vi "TL24 Tool Main.vi"() -> ()   [LabVIEW 2016]
uses:
  Common/LabVIEW GEA2 Toolkit/LabVIEW_GEA2_Toolkit.lvlibp/type defs/Data In.ctl
  Common/LabVIEW GEA2 Toolkit/LabVIEW_GEA2_Toolkit.lvlibp/type defs/Source_Destination.ctl
  Common/LabVIEW GEA2 Toolkit/LabVIEW_GEA2_Toolkit.lvlibp/type defs/Data Type.ctl
  Common/LabVIEW GEA2 Toolkit/LabVIEW_GEA2_Toolkit.lvlibp/type defs/ERD Read Data In.ctl
  Laundry Tool 2.0 Support/type defs2/Select _Graph_Brass.ctl
  Laundry Tool 1.0 Support/type defs/ERD_Graph_All.ctl
  Laundry Tool 1.0 Support/type defs/ERD_Graph.ctl
  Laundry Tool 1.0 Support/type defs/Version.ctl
  Laundry Tool 2.0 Support/type defs2/ERD_Always_Show_Brass.ctl
  Laundry Tool 1.0 Support/type defs/Fault_Buffer_Status.ctl
  Laundry Tool 2.0 Support/type defs2/Diagnostics_Table.ctl
  Laundry Tool 1.0 Support/type defs/Cycle_Diag_Buffer_Status.ctl
  Laundry Tool 2.0 Support/type defs2/ERD_Data_Loop_Control_Brass.ctl
  Laundry Tool 2.0 Support/type defs2/ERD_Loop_States_Brass.ctl
  Laundry Tool 2.0 Support/type defs2/Error_Command_Brass.ctl
  Laundry Tool 2.0 Support/type defs2/DAQ_States_Brass.ctl
  Common/GExplorer Support/typedefs/GExplorer_Data_Cluster.ctl
  Laundry Tool 1.0 Support/type defs/Cont_Send_States.ctl
  Laundry Tool 2.0 Support/type defs2/Cont_Send_States_Brass.ctl
  Common/LabVIEW GEA2 Toolkit/LabVIEW_GEA2_Toolkit.lvlibp/type defs/Data Out.ctl
  Common/LabVIEW GEA2 Toolkit/LabVIEW_GEA2_Toolkit.lvlibp/type defs/ERD Write Data In.ctl
  Laundry Tool 2.0 Support/type defs2/DAQ_Control_Command_Brass.ctl
  Laundry Tool 2.0 Support/type defs2/ERD_Loop_Control_Command_Brass.ctl
  Laundry Tool 2.0 Support/type defs2/GEA2_Control_Command_Brass.ctl
  <vilib>/DAQmx/read.llb/DAQmx Read (Digital 1D Bool NChan 1Samp 1Line).vi
  <vilib>/DAQmx/read.llb/DAQmx Read (Digital 1D U8 1Chan NSamp).vi
  <vilib>/DAQmx/write.llb/DAQmx Write (Digital Bool 1Line 1Point).vi
  <vilib>/DAQmx/read.llb/DAQmx Read (Counter U32 1Chan 1Samp).vi
  <vilib>/DAQmx/write.llb/DAQmx Write (Analog 1D DBL NChan 1Samp).vi
  <vilib>/DAQmx/write.llb/DAQmx Write (Digital 1D Bool NChan 1Samp 1Line).vi
  Common/LabVIEW GEA2 Toolkit/LabVIEW_GEA2_Toolkit.lvlibp/advanced/GEA2 Message Received Event Handler.vi
  <vilib>/DAQmx/create/channels.llb/DAQmx Create Channel (DO-Digital Output).vi
  <vilib>/DAQmx/create/channels.llb/DAQmx Create Channel (DI-Digital Input).vi
  <vilib>/DAQmx/configure/timing.llb/DAQmx Timing (Sample Clock).vi
  <vilib>/DAQmx/create/channels.llb/DAQmx Create Channel (CO-Pulse Generation-Frequency).vi
  <vilib>/DAQmx/configure/timing.llb/DAQmx Timing (Implicit).vi
  <vilib>/DAQmx/create/channels.llb/DAQmx Create Channel (CI-Count Edges).vi
  <vilib>/DAQmx/create/channels.llb/DAQmx Create Channel (AO-Voltage-Basic).vi
  <vilib>/DAQmx/miscellaneous.llb/DAQmx Fill In Error Info.vi
  C:/Automation/DLLs/PC Dot Net/GeaCommunication.dll
  Common/LabVIEW GEA2 Toolkit/LabVIEW_GEA2_Toolkit.lvlibp
  Automation/Product Specific/Clothes Care/2015 VA Washer/Projects/2015 VA Washer.lvlib
  <resource>/objmgr/daqmx.rc
panel:
  in  "Data ON":bool=TRUE
  out "ERD_Always Show":T1
  in  "Stop":bool
  out "Fault Status":bool
  out "Log Rate (ms)":u32
  in  "Tab Control":T2(tab)
  in  "Filter Data":bool=TRUE
  in  "Start Send":bool
  in  "Cmd":string
  in  "Filter Log":bool
  in  "Msg Rate (ms)":u32=1000 min=50 step=50
  out "CSV File Log Path":path=path "C:/Users/502129737/Desktop/1"
  in  "Clear":bool
  out "GEA2 Log":string
  in  "Board Index":u8 max=0 step=1
  out "Board ID":string="0"
  in  "GEA2 Send":T3={"Source"=228, "Destination"=50, "Command"=0, "Message"=""} {"Command" format="%02x"; "Destination" format="%02x"; "Source" format="%02x"}
  in  "Send Button":bool
  in  "GEA2 Log Length":i32=100000
  in  "Save Log":bool
  out "Version":T4
  in  "GEA Inputs":T5={"Source"=228, "Destination"=50} {"Destination" format="%.0x"; "Source" format="%.0x"}
  in  "Read ERD List":T6[](array[typedef])=[{"ERD Number"=0, "Data Type"=enum."string"}] {"ERD Number" format="%.0x"}
  out "Read ERD Data Out":cluster{"ERD Number":u16, "Data":string}[](array[cluster]) {"ERD Number" format="%.0x"}
  in  "Read ERD":bool
  in  "Write ERD":bool
  in  "Write ERD List":T8(array[cluster])=[{"ERD Number"=0, "Data Type"=enum."string", "Data"=""}] {"ERD Number" format="%.0x"}
  in  "ERD Graphing ON":bool
  out "ERD Graph  Ind":T9
  in  "ERD Graph Cntrl":T10={"ERD 3"={"ERD #"=62250, "Data Type"=enum."uint16_t", "Scaler"=32}, "ERD 2"={"ERD #"=62250, "Data Type"=enum."uint16_t", "Scaler"=32}, "ERD 1"={"ERD #"=62250, "Data Type"=enum."uint16_t", "Scaler"=32}} {"ERD 1"."Scaler" min=1; "ERD 1"."ERD #" format="%.0x"; "ERD 2"."Scaler" min=1; "ERD 2"."ERD #" format="%.0x"; "ERD 3"."Scaler" min=1; "ERD 3"."ERD #" format="%.0x"}
  in  "Graphing ON":bool=TRUE
  in  "Select Graph":T12=enum."All Loads"
  out "ERD 3":dbl(graph)
  out "ERD 2":dbl(graph)
  out "ERD 1":dbl(graph)
  in  "Save Fault Log":bool
  in  "Clear Fault Table Buffer":bool
  in  "Clear Fault Seq Buffer":bool
  in  "Fault ON":bool
  out "Fault Table Buffer":string[][](table)
  out "Fault Sequence Buffer":string
  out "Seq Buffer Status":T13
  out "Table Buffer Status":T13
  in  "Save Cycle History Log":bool
  in  "Clear Cycle Buffer":bool
  out "Cycle Buffer Status":T14
  in  "Get Cycle History":bool
  out "Diagnostics Table":T15
  in  "HE/LE ?":enum16{"HE", "LE"}(ring)
  in  "LL (M - A)":bool=TRUE
  in  "Lid Lock Feedback":bool
  in  "MS (M - A)":bool=TRUE
  out "DAQ Status":string
  out "Drain Pump":bool
  out "Mode Shift":bool
  out "Recirc Pump":bool
  out "Cold Valve":bool
  out "Hot Valve":bool
  out "Spray/Rinse Valve":bool
  out "Fabric SoftValve":bool
  in  "AC Power":bool=TRUE
  in  "Mode Shift FB":bool
  in  "Lid Status":bool=TRUE
  in  "Pressure":dbl(slide) min=0.0 max=5.0 step=0.5 scale=0.0..5.0 scale format="%#_3g"
  in  "Motor Current":dbl(slide)=2.5 min=0.0 max=5.0 step=0.5 scale=0.0..5.0 scale format="%#_3g"
  in  "Turn On DAQ":bool
  out "DAQ On?":bool
  in  "Basket RPM":dbl=1.0 min=1.0 max=800.0 step=5.0
  in  "Temperature":dbl(slide)=2.5 min=0.0 max=5.0 step=0.5 scale=0.0..5.0 scale format="%#_3g"
  out "Triac CW":bool
  out "Traic CCW":bool
  out "CCW":u32
  out "CW":u32
  in  "ERD Read List":T16(array[cluster])=[{"Boolean"=TRUE, "ERD Number"=1, "ERD Name"="Model Number", "Data Type"=enum."string"}, {"Boolean"=TRUE, "ERD Number"=2, "ERD Name"="Serial Number", "Data Type"=enum."string"}, {"Boolean"=TRUE, "ERD Number"=8192, "ERD Name"="Machine Status", "Data Type"=enum."uint8_t"}, {"Boolean"=TRUE, "ERD Number"=8202, "ERD Name"="Cycle Name", "Data Type"=enum."string"}, {"Boolean"=TRUE, "ERD Number"=8213, "ERD Name"="Soil Level", "Data Type"=enum."string"}, {"Boolean"=TRUE, "ERD Number"=142, "ERD Name"="Cycle Count", "Data Type"=enum."uint32_t"}, {"Boolean"=TRUE, "ERD Number"=8193, "ERD Name"="Sub-Cycle", "Data Type"=enum."string"}, {"Boolean"=TRUE, "ERD Number"=141, "ERD Name"="System Runtime", "Data Type"=enum."uint32_t"}, {"Boolean"=TRUE, "ERD Number"=8208, "ERD Name"="Delay Time", "Data Type"=enum."uint16_t"}, {"Boolean"=TRUE, "ERD Number"=256, "ERD Name"="Version", "Data Type"=enum."string"}, {"Boolean"=TRUE, "ERD Number"=70, "ERD Name"="Cycle Time", "Data Type"=enum."uint16_t"}, {"Boolean"=TRUE, "ERD Number"=8206, "ERD Name"="Operating Mode", "Data Type"=enum."string"}, {"Boolean"=TRUE, "ERD Number"=8214, "ERD Name"="Temp Level", "Data Type"=enum."uint8_t"}, {"Boolean"=TRUE, "ERD Number"=8215, "ERD Name"="Spin Level", "Data Type"=enum."uint8_t"}, {"Boolean"=TRUE, "ERD Number"=61440, "ERD Name"="Water Level", "Data Type"=enum."uint8_t"}, {"Boolean"=TRUE, "ERD Number"=8216, "ERD Name"="Rinse Option", "Data Type"=enum."uint8_t"}] {"ERD Number" format="%.0x"}
  out "Error Out":errorcluster
  in  "Error In":errorcluster
  # "Software Version"
  # "UI"
  # "MC"
  # "Must input a valid ERD# and Data Type\nDO NOT Leave Blank \nIf no scaler use value of 01"
  # "Contact:\n\nDerek Hibdon\nderek.hibdon@ge.com"
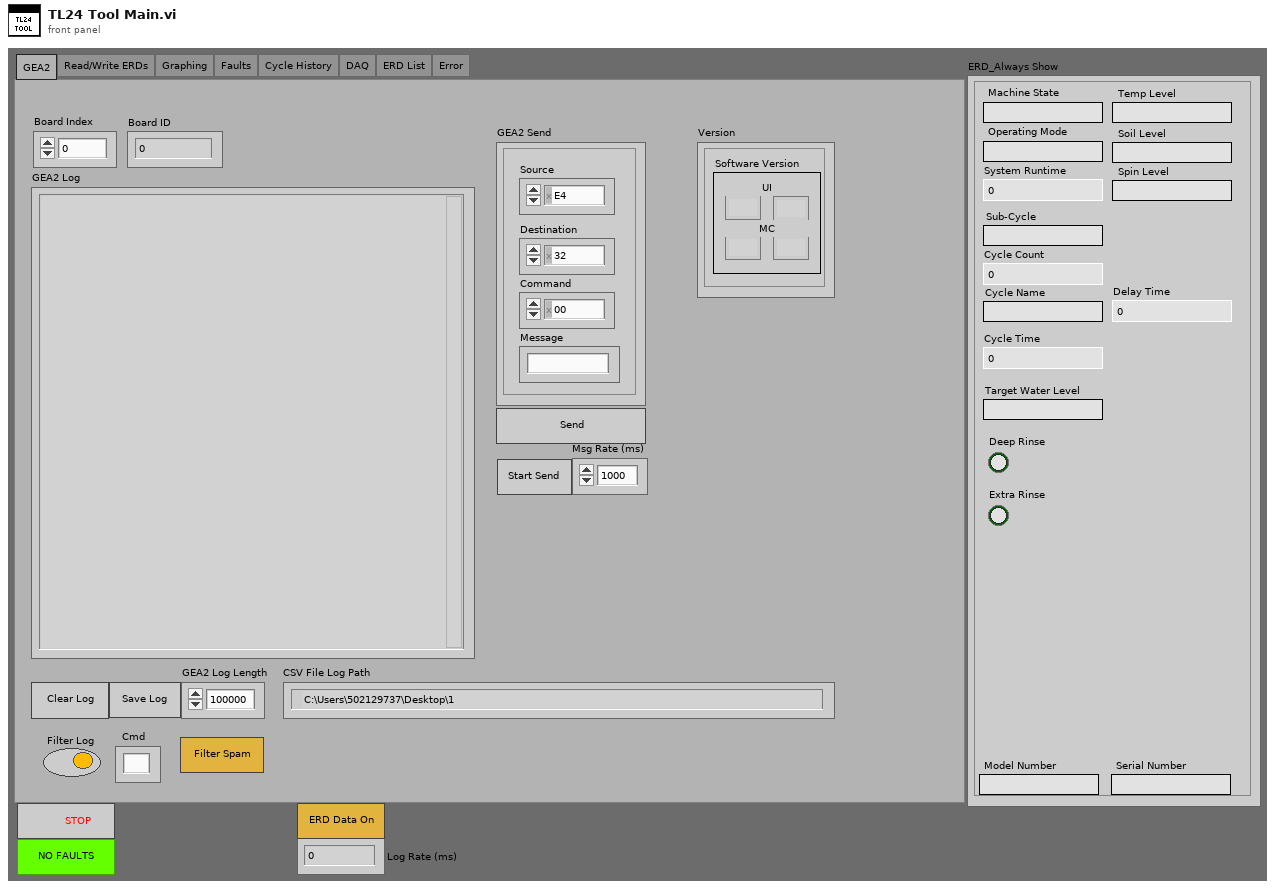
[diagram p1: front panel]
types:
  T1 = typedef "ERD_Always_Show_Brass.ctl" = cluster{"Machine State":string, "Cycle Count":u32, "Soil Level":string, "Spin Level":string, "Temp Level":string, "Delay Time":u16, "Sub-Cycle":string, "Cycle Name":string, "Model Number":string, "Serial Number":string, "System Runtime":u32, "Cycle Time":u16, "Operating Mode":string, "Target Water Level":string, "Deep Rinse":bool, "Extra Rinse":bool}
  T2 = enum32{"GEA2", "Read/Write ERDs", "Graphing", "Faults", "Cycle History", "DAQ", "ERD List", "Error"}
  T3 = typedef "LabVIEW_GEA2_Toolkit.lvlibp/Data In.ctl" = cluster{"Source":u8, "Destination":u8, "Command":u8, "Message":string}
  T4 = typedef "Version.ctl" = cluster{"Critical Major":string, "Critical Minor":string, "Non-Critical Minor":string, "Non-Critical Major":string}
  T5 = typedef "LabVIEW_GEA2_Toolkit.lvlibp/Source_Destination.ctl" = cluster{"Source":u8, "Destination":u8}
  T6 = typedef "LabVIEW_GEA2_Toolkit.lvlibp/ERD Read Data In.ctl" = cluster{"ERD Number":u16, "Data Type":T7}
  T7 = typedef "LabVIEW_GEA2_Toolkit.lvlibp/Data Type.ctl" = enum16{"string", "boolean", "uint8_t", "uint16_t", "uint32_t", "uint64_t", "int8_t", "int16_t", "int32_t", "int64_t"}
  T8 = cluster{"ERD Number":u16, "Data Type":T7, "Data":string}[]
  T9 = cluster{"ERD Value 1":dbl, "ERD Value 2":dbl, "ERD Value 3":dbl}
  T10 = typedef "ERD_Graph_All.ctl" = cluster{"ERD 3":T11, "ERD 2":T11, "ERD 1":T11}
  T11 = typedef "ERD_Graph.ctl" = cluster{"ERD #":u16, "Data Type":T7, "Scaler":u32}
  T12 = typedef "Select _Graph_Brass.ctl" = enum16{"Temperature (F)", "Basket Speed (RPM)", "Tub Volume (Gal)", "Pressure (in H2O)", "Current RMS (Amps)", "ERD 1", "ERD 2", "ERD 3", "All Loads"}
  T13 = typedef "Fault_Buffer_Status.ctl" = cluster{"Current Index":u16, "Count":u16, "Overwrite Count":u16}
  T14 = typedef "Cycle_Diag_Buffer_Status.ctl" = cluster{"Current Index":u16, "Count":u16, "Overwrite Count":u16}
  T15 = typedef "Diagnostics_Table.ctl" = string[][]
  T16 = cluster{"Boolean":bool, "ERD Number":u16, "ERD Name":string, "Data Type":enum16{"string", "boolean", "uint8_t", "uint16_t", "uint32_t", "uint64_t"}}[]
  T17 = typedef "Cont_Send_States_Brass.ctl" = enum16{"Run", "Shutdown"}
  T18 = typedef "Cont_Send_States.ctl" = enum16{"Run", "Shutdown"}
  T19 = typedef "GExplorer_Data_Cluster.ctl" = cluster{"Data":variant, "State":enum16{"Add to Log", "Clear", "Shutdown"}}
  T20 = typedef "DAQ_States_Brass.ctl" = enum16{"Wait for Init", "Rename Devices", "Verify Hardware", "Initialize", "Run", "Shutdown", "Exit"}
  T21 = typedef "ERD_Data_Loop_Control_Brass.ctl" = cluster{"Data":variant, "State":T22}
  T22 = typedef "ERD_Loop_States_Brass.ctl" = enum16{"Init", "Build ERD Read List", "Read ERDs", "Update UI", "Update Graphs", "Read Faults", "Log Data", "Pause", "Shutdown"}
  T23 = typedef "Error_Command_Brass.ctl" = enum16{"Initialize", "Handle Errors", "Report Errors"}
  T24 = typedef "LabVIEW_GEA2_Toolkit.lvlibp/ERD Write Data In.ctl" = cluster{"ERD Number":u16, "Data Type":T7, "Data":string}
  T25 = typedef "GEA2_Control_Command_Brass.ctl" = enum16{"Initialize", "Shutdown"}
  T26 = typedef "ERD_Loop_Control_Command_Brass.ctl" = enum16{"Initialize", "Shutdown"}
  T27 = typedef "DAQ_Control_Command_Brass.ctl" = enum16{"Initialize", "Shutdown", "Exit"}
  T28 = enum8{"Enabled", "Disabled", "Disabled and Grayed Out"}
  T29 = typedef "LabVIEW_GEA2_Toolkit.lvlibp/Data Out.ctl" = cluster{"Source":u8, "Destination":u8, "Command":u8, "Length":u8, "CRC":u16, "Message":string}
  T30 = typedef "LabVIEW_GEA2_Toolkit.lvlibp/ERD Read Data Out.ctl" = cluster{"ERD Number":u16, "Data":string}
  T31 = typedef "All_Bundled_Data_Brass.ctl" = cluster{"Version":T4, "ERD_Always Show":T1, "Personality Set":u8, "CSV File String Arrays":T32, "Fault Table Array ":T33}
  T32 = typedef "CSV_File_String_Arrays.ctl" = cluster{"ERD Number Array":string[], "ERD Name Array":string[], "ERD Converted String Data":string[]}
  T33 = typedef "Fault Table Array.ctl" = T34[]
  T34 = typedef "Fault_Table_Info.ctl" = cluster{"Cycle Count":u32, " Runtime (min) ":u32, "Fault Status":string, "Fault ID":string, "Fault Count":u16}
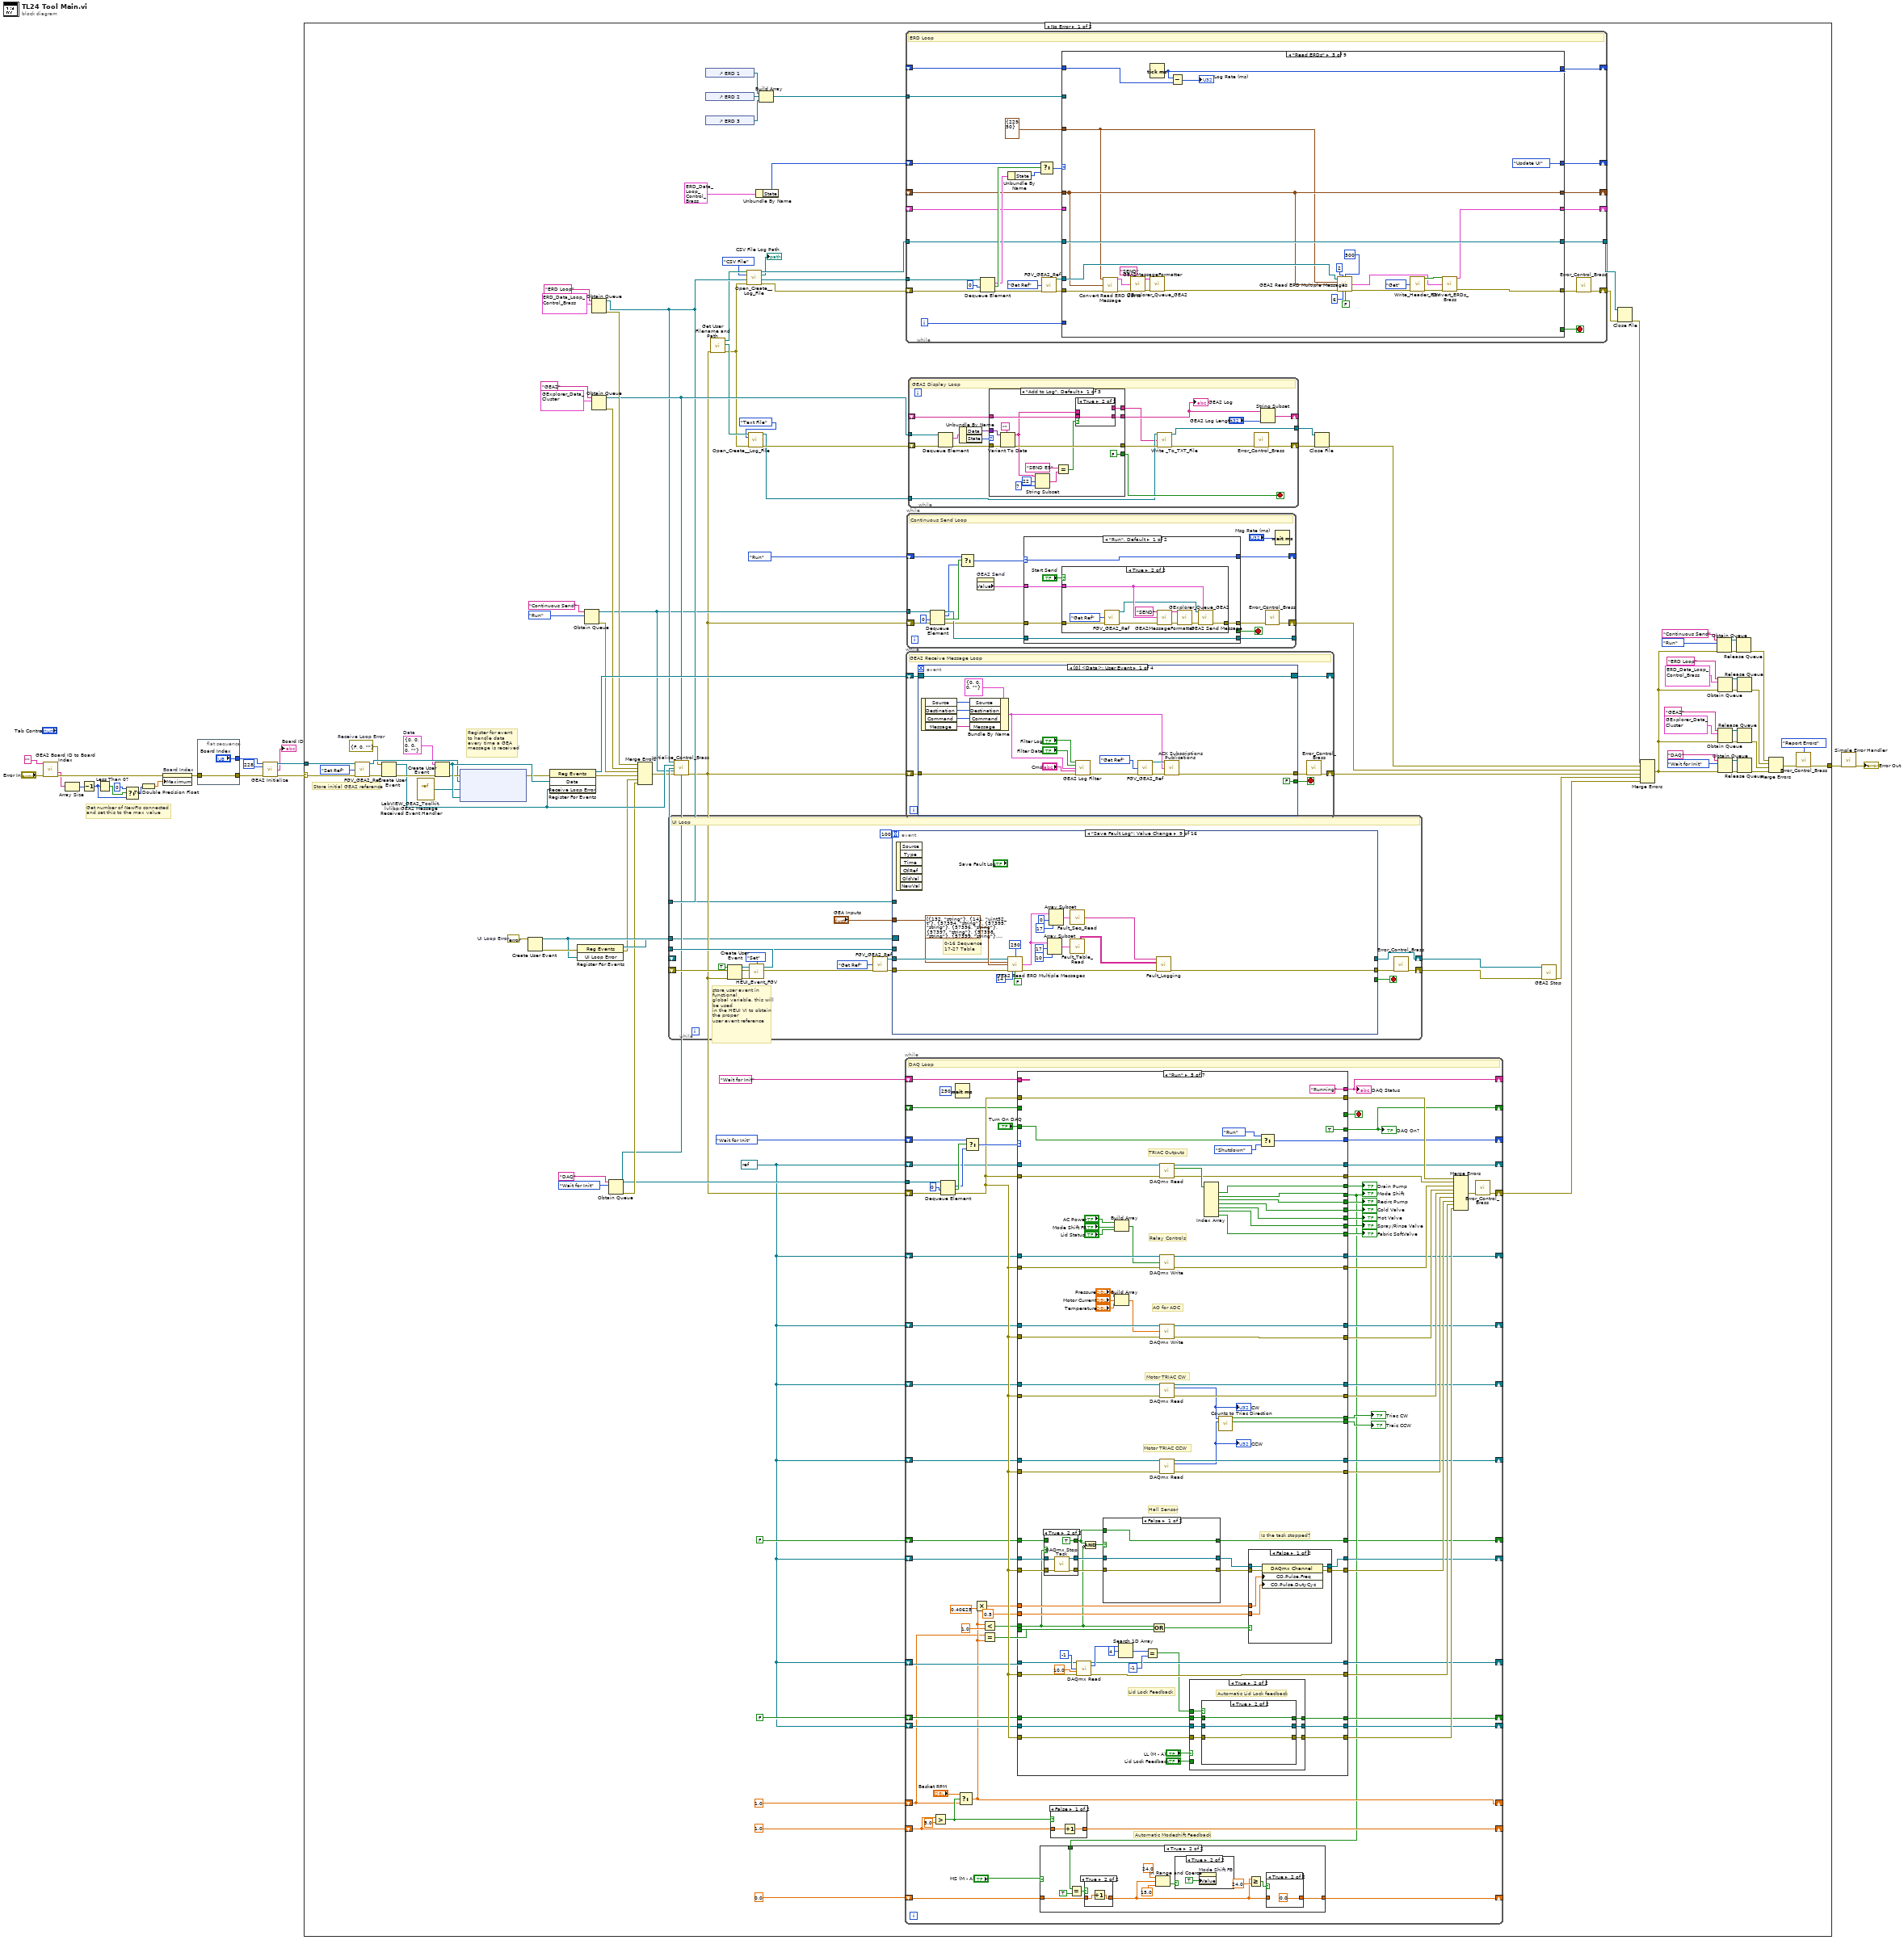
[diagram p0: block diagram]
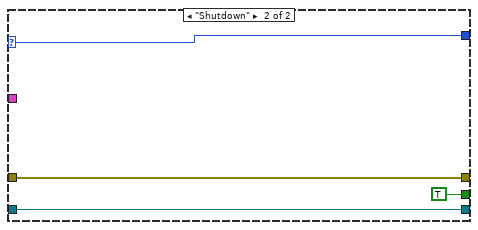
[diagram p3: hidden frame]
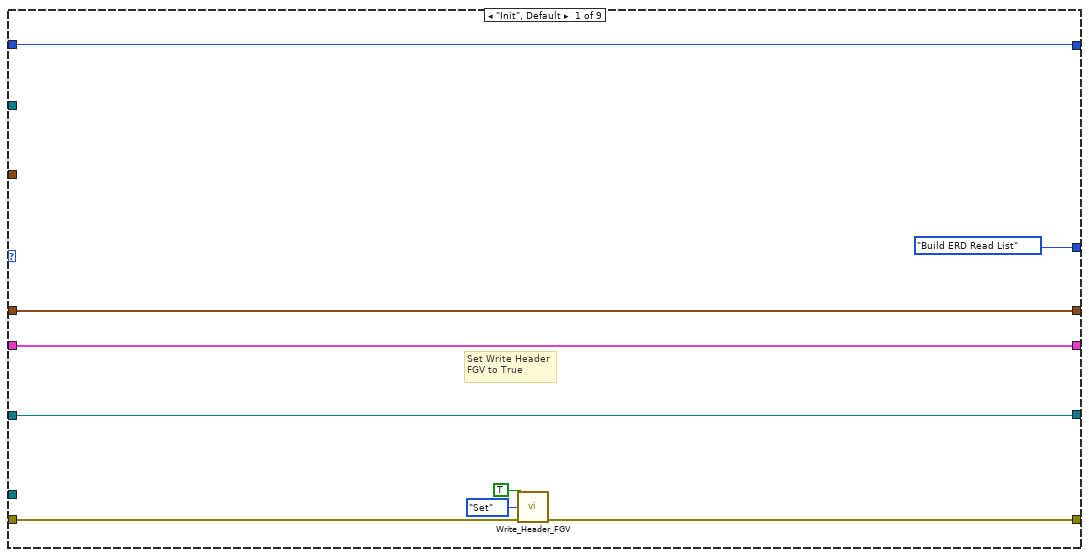
[diagram p4: hidden frame]
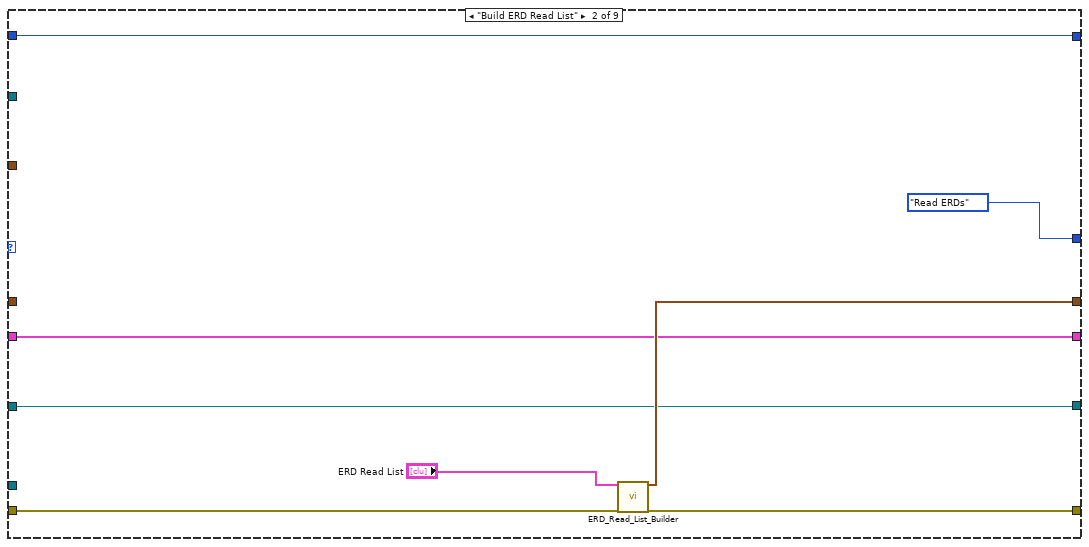
[diagram p5: hidden frame]
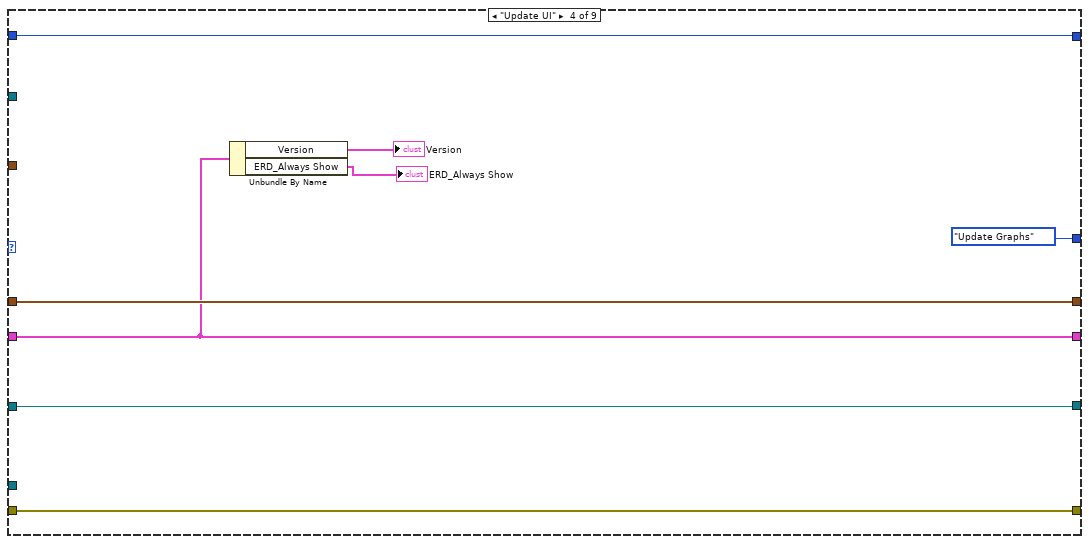
[diagram p6: hidden frame]
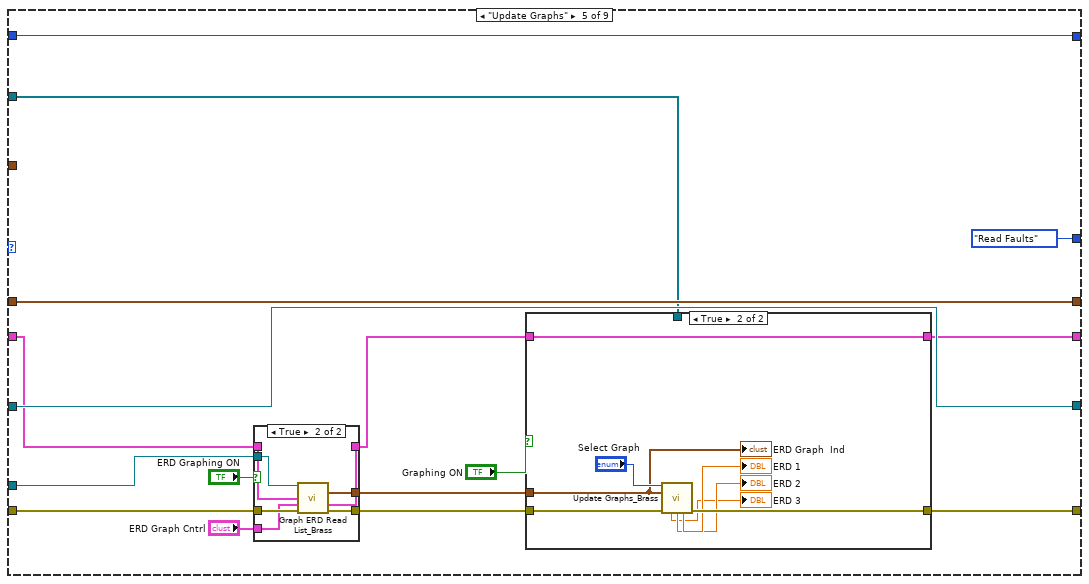
[diagram p7: hidden frame]
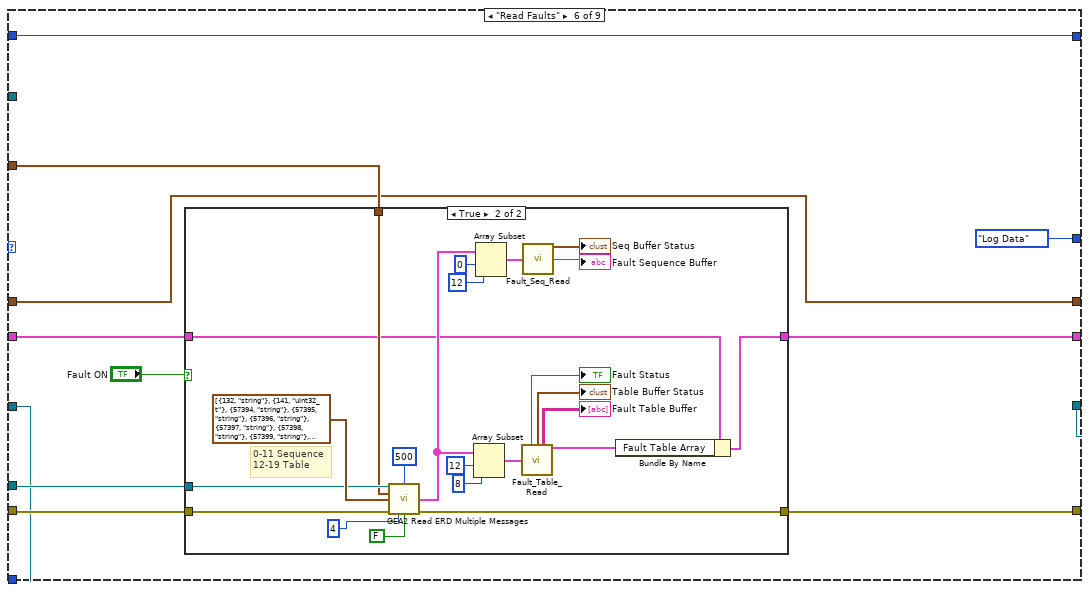
[diagram p10: hidden frame]
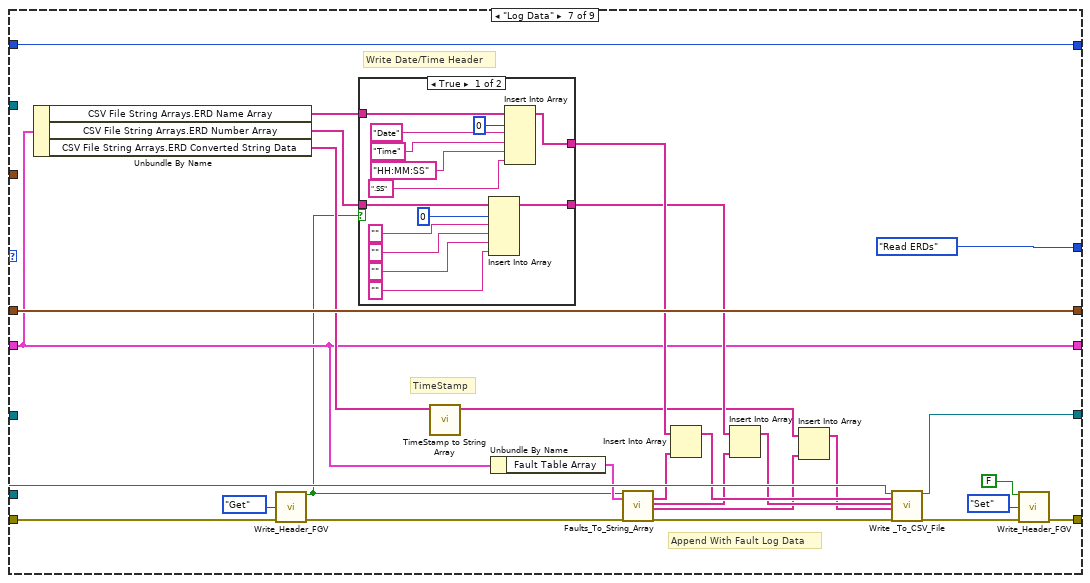
[diagram p12: hidden frame]
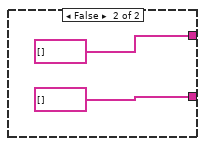
[diagram p13: hidden frame]
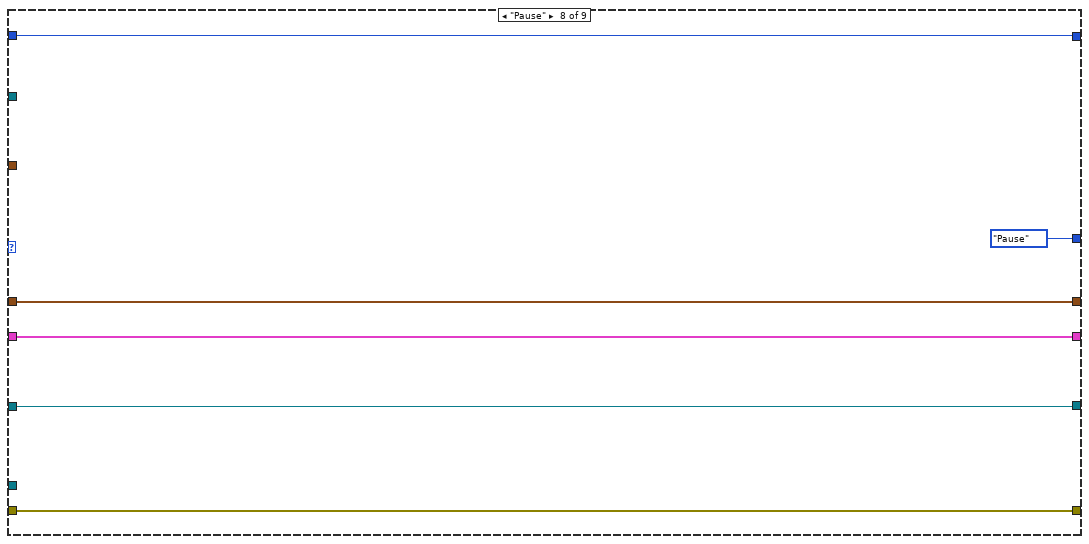
[diagram p14: hidden frame]
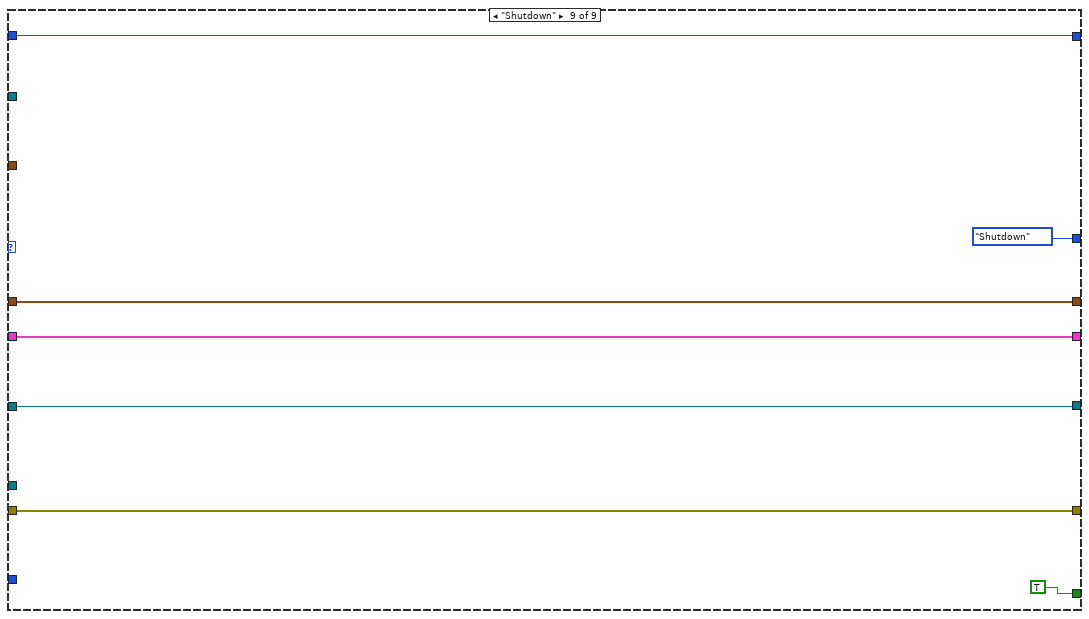
[diagram p15: hidden frame]
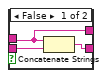
[diagram p16: hidden frame]
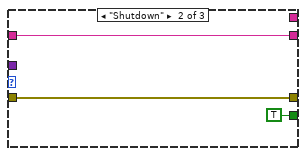
[diagram p17: hidden frame]
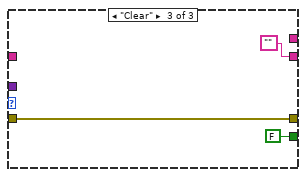
[diagram p18: hidden frame]
diagram:
  # "Get number of NewFIs connected\nand set this to the max value"
  n1 = call "GEA2 Board ID to Board Index.vi"("Board ID"="", "Error In"="Error In") -> ("Boards Found"=w4:string[], "Error Out"=w13:errorcluster)  [unwired: 9 in, 3 out]
  n2 = Array Size(array=w4) -> (size(s)=w9:i32)
  n3 = Decrement(x=w9) -> (x-1=w7:i32)
  n4 = Less Than 0?(x=w7) -> (x < 0?=w8:bool)
  n5 = Select(t=0, s=w8, f=w7) -> (s? t:f=w5:i32)
  n6 = To Double Precision Float(number=w5) -> (double precision float=w3:dbl)
  n7 = property on="Board Index" class="DigNum (strict)"(error in=w13, "Maximum"=w3) -> (error out=w11:errorcluster)  [unwired: 1 in, 1 out]
  n8 = flat-sequence {
    tunnel: ["Board Index"] -> w16
    tunnel: w11 -> [w20]
    tunnel: [w20] -> w10
    frame #0 {
    }
  }
  n9 = call "GEA2 Initialize.vi"("Board Index"=w16, "Source Address"=u8 228, "error in"=w10) -> ("GEA2 Reference Out"=w18:refnum<k24>, "Board ID"=→"Board ID":string, "error out"=w17:errorcluster)  [unwired: 10 in]
  n10 = case shown="No Error" w17 {
    selector: w17 -> [w80 w1258]
    tunnel: w18 -> [w78 _]
    tunnel: [w82 w1258] -> w2
    frame No Error {
      w34 = errorcluster {"status"=FALSE, "code"=0, "source"=""}  # Receive Loop Error
      w35 = T29 {"Source"=0, "Destination"=0, "Command"=0, "Length"=0, "CRC"=0, "Message"=""}  # Data
      w50 = refnum<k21> refnum ("task out")
      w116 = errorcluster {"status"=FALSE, "code"=0, "source"=""}  # UI Loop Error
      # "store user event in functional\nglobal variable, this will be used\nin the HEUI VI to obtain the proper\nuser event reference"
      # "Store initial GEA2 reference"
      # "Register for event\nto handle data\nevery time a GEA\nmessage is received"
      n11 = call "FGV_GEA2_Ref.vi"("GEA2 Reference In"=w78, "Action"=enum16{"Set Ref", "Get Ref"}."Set Ref", "Error In"=w80) -> ("GEA2 Reference Out"=w77:refnum<k24>, "Error Out"=w79:errorcluster)  [unwired: 11 in]
      n12 = Create User Event(user event datatype=w34, error in=w79) -> (user event=w117:refnum<user-event>, error out=w119:errorcluster)
      n13 = vi-ref "LabVIEW_GEA2_Toolkit.lvlibp:GEA2 Message Received Event Handler.vi"() -> (w118:refnum<vi>)
      n14 = Create User Event(user event datatype=w35, error in=w119) -> (user event=w122:refnum<user-event>, error out=w121:errorcluster)
      n15 = node(w121, w77, w118, w122) -> (w120:errorcluster)  [unwired: 1 in, 1 out]
      n16 = Create User Event(user event datatype=w116) -> (user event=w105:refnum<user-event>, error out=w115:errorcluster)  [unwired: 1 in]
      n17 = register-events(error in=w120, w122, w117) -> (reference out=w114:refnum<event-registration>, error out=w87:errorcluster)  [unwired: 1 in]
      n18 = register-events(error in=w115, w105) -> (reference out=w96:refnum<event-registration>, error out=w86:errorcluster)  [unwired: 1 in]
      n19 = Obtain Queue(name (unnamed)="Continuous Send", element data type=Cont_Send_States_Brass."Run" ("State")) -> (queue out=w36:refnum<queue>, error out=w41:errorcluster)  [unwired: 3 in, 1 out]
      n20 = Obtain Queue(name (unnamed)="ERD Loop", element data type=T21 {"Data"=variant, "State"=enum."Read ERDs"} ("Data")) -> (queue out=w65:refnum<queue>, error out=w83:errorcluster)  [unwired: 3 in, 1 out]
      n21 = Obtain Queue(name (unnamed)="GEA2", element data type=T19 {"Data"=variant, "State"=enum."Add to Log"} ("Data")) -> (queue out=w66:refnum<queue>, error out=w88:errorcluster)  [unwired: 3 in, 1 out]
      n22 = Obtain Queue(name (unnamed)="DAQ", element data type=DAQ_States_Brass."Wait for Init" ("States")) -> (queue out=w58:refnum<queue>, error out=w85:errorcluster)  [unwired: 3 in, 1 out]
      n23 = Merge Errors(w83, w88, w41, w87, w86, w85) -> (w84:errorcluster)
      n24 = call "Initialize_Control_Brass.vi"("ERD Loop"=w65, "GEA2"=w66, "Receive Loop"=w117, "UI Loop Error"=w105, "Cont Send"=w36, "Error In"=w84, "DAQ"=w58) -> ("Error Out"=w31:errorcluster)  [unwired: 8 in]
      n25 = control-ref of="ERD 1"() -> (w62:refnum<vi>)
      n26 = control-ref of="ERD 2"() -> (w60:refnum<vi>)
      n27 = control-ref of="ERD 3"() -> (w61:refnum<vi>)
      n28 = call "Get User Filename and Path.vi"("error in (no error)"=w31) -> ("error out"=w23:errorcluster, "TXT File Path"=w29:path, "CSV File Path"=w32:path)  [unwired: 8 in]
      n29 = Create User Event(user event datatype=TRUE ("Bool"), error in=w31) -> (user event=w72:refnum<user-event>, error out=w73:errorcluster)
      n30 = call "Open_Create__Log_File.vi"("File Path Control"=w32, "Enum"=enum16{"CSV File", "Text File"}."CSV File", "Error In"=w23) -> ("refnum out"=w63:refnum<file>, "File Path"=→"CSV File Log Path":path, "Error Out"=w75:errorcluster)  [unwired: 10 in]
      n31 = call "Open_Create__Log_File.vi"("File Path Control"=w29, "Enum"=enum16{"CSV File", "Text File"}."Text File", "Error In"=w23) -> ("refnum out"=w28:refnum<file>, "Error Out"=w30:errorcluster)  [unwired: 10 in, 1 out]
      n32 = call "HEUI_Event_FGV.vi"("Event In"=w72, "Action"=enum16{"Get", "Set"}."Set", "Error In"=w73) -> ("Event Out"=w69:refnum<user-event>, "Error Out"=w70:errorcluster)  [unwired: 11 in]
      n33 = while "UI Loop" {
        shift-right: [w1008] -> w124
        shift-left: w70 -> [w1002]
        shift-right: [w1010] -> w123
        shift-left: _ -> [_]
        tunnel: w96 -> [w1009]
        tunnel: w69 -> [w999]
        tunnel: w65 -> [w998]
        stop <- w1007 stop-if-true
        # "UI Loop"
        n34 = call "FGV_GEA2_Ref.vi"("Action"=enum16{"Set Ref", "Get Ref"}."Get Ref", "Error In"=w1002) -> ("GEA2 Reference Out"=w1001:refnum<k24>, "Error Out"=w1003:errorcluster)  [unwired: 12 in]
        n35 = event shown="[8] \"Save Fault Log\": Value Change" {
          selector: w1009 -> [_ _ _ _ _ _ _ _ _ _ _ _ _ _ _ _]
          dyn-events: _ -> [_ _ _ _ _ _ _ _ _ _ _ _ _ _ _ _]
          timeout: 100 -> [_ _ _ _ _ _ _ _ _ _ _ _ _ _ _ _]
          tunnel: [w1016 w1026 w1027 w1033 w1047 w1057 w1070 w1077 w1080 w1099 w1116 w1135 w1149 w1167 w1187 w1198] -> w1006
          tunnel: w1003 -> [w1013 w1023 w1027 w1029 w1044 w1061 w1068 w1075 w1084 w1102 w1119 w1141 w1157 w1173 w1188 w1205]
          tunnel: [_ _ _ _ _ _ _ _ _ _ _ _ _ _ _ TRUE] -> w1007
          tunnel: w1001 -> [w1011 w1025 w1028 w1031 w1045 _ _ _ w1086 w1101 w1118 w1140 w1151 w1172 _ w1208]
          tunnel: [w1018 w1025 w1028 w1034 w1046 _ _ _ _ w1100 w1117 _ _ _ _ w1208] -> w1010
          tunnel: "GEA Inputs" -> [_ _ _ w1032 w1042 _ _ _ w1085 w1103 w1120 w1138 w1150 w1174 _ _]
          tunnel: w999 -> [_ _ _ _ _ _ _ _ _ _ _ _ _ _ _ _]
          tunnel: w998 -> [_ _ _ _ _ _ w1066 w1073 _ _ _ _ _ _ w1185 _]
          event "Send Button": Value Change {
            n36 = event-data() -> ()  [unwired: 1 in, 1 out]
            n37 = call "GEA2MessageFormatter.vi"("Prefix(Send/Recv)"="SEND", "GEA2 Data In"="GEA2 Send", "Error In"=w1013) -> ("Output String"=w1015:string, "Error Out"=w1014:errorcluster)  [unwired: 11 in]
            n38 = call "GExplorer_Queue_GEA2.vi"("Output String"=w1015, "error in (no error)"=w1014) -> ("error out"=w1017:errorcluster)  [unwired: 13 in]
            n39 = call "GEA2 Send Message.vi"("GEA2 Reference In"=w1011, "Input Data"="GEA2 Send", "Error In"=w1017) -> ("GEA2 Reference Out"=w1018:refnum<k24>, "Error Out"=w1016:errorcluster)  [unwired: 11 in]
          }
          event "Clear": Value Change {
            w1020 = T19 {"Data"=variant, "State"=enum."Clear"} ("element")
            n40 = event-data() -> ()  [unwired: 1 in, 6 out]
            n41 = Obtain Queue(name (unnamed)="GEA2", element data type=w1020, error in (no error)=w1023) -> (queue out=w1021:refnum<queue>, error out=w1024:errorcluster)  [unwired: 2 in, 1 out]
            n42 = Enqueue Element(queue=w1021, element=w1020, error in (no error)=w1024) -> (error out=w1026:errorcluster)  [unwired: 1 in, 2 out]
          }
          event Timeout {
            # "Must have timeout case to give GEA2 FGV a chance to update\nthe GEA2 reference. Otherwise, when we receive an event it may\nbe using a reference that is no longer valid."
            n43 = event-data() -> ()  [unwired: 1 in, 3 out]
          }
          event "Write ERD": Value Change {
            n44 = event-data() -> ()  [unwired: 1 in, 1 out]
            n45 = call "Convert Write ERD List to Message.vi"("GEA Inputs"=w1032, "Write ERD List"="Write ERD List", "Error In"=w1029) -> ("GEA Message"=w1038:T3, "Error Out"=w1039:errorcluster)  [unwired: 11 in]
            n46 = call "GEA2MessageFormatter.vi"("Prefix(Send/Recv)"="SEND", "GEA2 Data In"=w1038, "Error In"=w1039) -> ("Output String"=w1040:string, "Error Out"=w1041:errorcluster)  [unwired: 11 in]
            n47 = call "GExplorer_Queue_GEA2.vi"("Output String"=w1040, "error in (no error)"=w1041) -> ("error out"=w1036:errorcluster)  [unwired: 13 in]
            n48 = call "GEA2 Write ERD.vi"("GEA2 Reference In"=w1031, "GEA Inputs"=w1032, "Write ERD List"="Write ERD List", "Error In"=w1036, "Verify ERD Response?"=FALSE) -> ("GEA2 Reference Out"=w1034:refnum<k24>, "Error Out"=w1033:errorcluster)  [unwired: 8 in, 1 out]
          }
          event "Read ERD": Value Change {
            n49 = event-data() -> ()  [unwired: 1 in, 6 out]
            n50 = call "Convert Read ERD List to Message.vi"("GEA Inputs"=w1042, "Read ERD List"="Read ERD List", "Error In"=w1044) -> ("GEA Message"=w1052:T3, "Error Out"=w1043:errorcluster)  [unwired: 11 in]
            n51 = call "GEA2MessageFormatter.vi"("Prefix(Send/Recv)"="SEND", "GEA2 Data In"=w1052, "Error In"=w1043) -> ("Output String"=w1050:string, "Error Out"=w1049:errorcluster)  [unwired: 11 in]
            n52 = call "GExplorer_Queue_GEA2.vi"("Output String"=w1050, "error in (no error)"=w1049) -> ("error out"=w1053:errorcluster)  [unwired: 13 in]
            n53 = call "GEA2 Read ERD.vi"("GEA2 Reference In"=w1045, "GEA Inputs"=w1042, "Read ERD List"="Read ERD List", "Error In"=w1053, "Verify ERD Response?"=FALSE) -> ("GEA2 Reference Out"=w1046:refnum<k24>, "ERD Data Out"=→"Read ERD Data Out":T30[], "Error Out"=w1047:errorcluster)  [unwired: 7 in, 1 out]
          }
          event "Save Log": Value Change {
            n54 = event-data() -> ()  [unwired: 1 in, 6 out]
            n55 = property on="GEA2 Log" class="Str"(error in=w1061) -> (error out=w1063:errorcluster, "Value"=w1062:string)  [unwired: 1 in, 1 out]
            n56 = Write to Text File(prompt (Choose or enter file path)="Choose filename and path to save txt file to ", text=w1062, error in=w1063) -> (refnum out=w1060:refnum<file>, error out=w1059:errorcluster)  [unwired: 1 in, 1 out]
            n57 = Close File(refnum=w1060, error in=w1059) -> (error out=w1058:errorcluster)  [unwired: 1 out]
            n58 = call <vilib>:"Clear Errors.vi"("error in (no error)"=w1058, "specific error code to clear (0: all)"=43) -> ("error out"=w1057:errorcluster)  [unwired: 4 in, 1 out]
          }
          event "ERD Read List": Value Change {
            n59 = event-data() -> ()  [unwired: 1 in, 6 out]
            n60 = Enqueue Element(queue=w1066, element=T21 {"Data"=variant, "State"=enum."Build ERD Read List"}, error in (no error)=w1068) -> (error out=w1067:errorcluster)  [unwired: 1 in, 2 out]
            n61 = call "Write_Header_FGV.vi"("Write Header ? In"=TRUE, "Action"=enum16{"Get", "Set"}."Set", "Error In"=w1067) -> ("Error Out"=w1070:errorcluster)  [unwired: 11 in, 1 out]
          }
          event "Fault ON", "ERD Graphing ON": Value Change {
            n62 = event-data() -> ()  [unwired: 1 in, 6 out]
            n63 = Enqueue Element(queue=w1073, element=T21 {"Data"=variant, "State"=enum."Build ERD Read List"}, error in (no error)=w1075) -> (error out=w1074:errorcluster)  [unwired: 1 in, 2 out]
            n64 = call "Write_Header_FGV.vi"("Write Header ? In"=TRUE, "Action"=enum16{"Get", "Set"}."Set", "Error In"=w1074) -> ("Error Out"=w1077:errorcluster)  [unwired: 11 in, 1 out]
          }
          event "Save Fault Log": Value Change {
            # "0-16 Sequence\n17-27 Table"
            n65 = event-data() -> ()  [unwired: 1 in, 6 out]
            n66 = call "GEA2 Read ERD Multiple Messages.vi"("GEA2 Reference In"=w1086, "Read Timeout (ms)"=u32 250, "GEA Inputs"=w1085, "Read ERD List"=T6[] [{"ERD Number"=132, "Data Type"=enum."string"}, {"ERD Number"=141, "Data Type"=enum."uint32_t"}, {"ERD Number"=57394, "Data Type"=enum."string"}, {"ERD Number"=57395, "Data Type"=enum."string"}, {"ERD Number"=57396, "Data Type"=enum."string"}, {"ERD Number"=57397, "Data Type"=enum."string"}, {"ERD Number"=57398, "Data Type"=enum."string"}, {"ERD Number"=57399, "Data Type"=enum."string"}, {"ERD Number"=57400, "Data Type"=enum."string"}, {"ERD Number"=57401, "Data Type"=enum."string"}, {"ERD Number"=57402, "Data Type"=enum."string"}, {"ERD Number"=57403, "Data Type"=enum."string"}, {"ERD Number"=57404, "Data Type"=enum."string"}, {"ERD Number"=57405, "Data Type"=enum."string"}, {"ERD Number"=57406, "Data Type"=enum."string"}, {"ERD Number"=57407, "Data Type"=enum."string"}, {"ERD Number"=57408, "Data Type"=enum."string"}, {"ERD Number"=129, "Data Type"=enum."string"}, {"ERD Number"=57444, "Data Type"=enum."string"}, {"ERD Number"=57445, "Data Type"=enum."string"}, {"ERD Number"=57446, "Data Type"=enum."string"}, {"ERD Number"=57447, "Data Type"=enum."string"}, {"ERD Number"=57448, "Data Type"=enum."string"}, {"ERD Number"=57449, "Data Type"=enum."string"}, {"ERD Number"=57450, "Data Type"=enum."string"}, {"ERD Number"=57451, "Data Type"=enum."string"}, {"ERD Number"=57452, "Data Type"=enum."string"}, {"ERD Number"=57453, "Data Type"=enum."string"}], "Error In"=w1084, "#ERDs per message"=14 ("#ERDs per message 2"), "Verify ERD Response?"=FALSE) -> ("ERD Data Out"=w1089:T30[], "Error Out"=w1081:errorcluster)  [unwired: 5 in, 2 out]
            n67 = Array Subset(array=w1089, index=17, length=10) -> (w1090:T30[])
            n68 = Array Subset(array=w1089, index=0, length=17) -> (w1088:T30[])
            n69 = call "Fault_Seq_Read.vi"("Seq ERD In"=w1088) -> ("String"=w1083:string)  [unwired: 13 in, 1 out]
            n70 = call "Fault_Table_Read.vi"("ERD Data Out"=w1090) -> ("Fault Table String Out"=w1082:string[][])  [unwired: 11 in, 3 out]
            n71 = call "Fault_Logging.vi"("String"=w1083, "Fault Table String Out"=w1082, "error in (no error)"=w1081) -> ("error out"=w1080:errorcluster)  [unwired: 12 in]
          }
          event "Clear Fault Seq Buffer": Value Change {
            n72 = event-data() -> ()  [unwired: 1 in, 6 out]
            n73 = Bundle By Name(cluster=T24 {"ERD Number"=133, "Data Type"=enum."string", "Data"=""} ("ERD Read Data In"), "Data"="FF") -> (w1112:T24)
            n74 = Build Array(w1112) -> (w1106:T24[])
            n75 = call "Convert Write ERD List to Message.vi"("GEA Inputs"=w1103, "Write ERD List"=w1106, "Error In"=w1102) -> ("GEA Message"=w1108:T3, "Error Out"=w1109:errorcluster)  [unwired: 11 in]
            n76 = call "GEA2MessageFormatter.vi"("Prefix(Send/Recv)"="SEND", "GEA2 Data In"=w1108, "Error In"=w1109) -> ("Output String"=w1110:string, "Error Out"=w1111:errorcluster)  [unwired: 11 in]
            n77 = call "GExplorer_Queue_GEA2.vi"("Output String"=w1110, "error in (no error)"=w1111) -> ("error out"=w1107:errorcluster)  [unwired: 13 in]
            n78 = call "GEA2 Write ERD.vi"("GEA2 Reference In"=w1101, "Read Timeout (ms)"=u32 2000, "GEA Inputs"=w1103, "Write ERD List"=w1106, "Error In"=w1107, "Verify ERD Response?"=FALSE) -> ("GEA2 Reference Out"=w1100:refnum<k24>, "Error Out"=w1099:errorcluster)  [unwired: 7 in, 1 out]
          }
          event "Clear Fault Table Buffer": Value Change {
            n79 = event-data() -> ()  [unwired: 1 in, 6 out]
            n80 = Bundle By Name(cluster=T24 {"ERD Number"=130, "Data Type"=enum."string", "Data"=""} ("ERD Read Data In"), "Data"="FF") -> (w1129:T24)
            n81 = Build Array(w1129) -> (w1123:T24[])
            n82 = call "Convert Write ERD List to Message.vi"("GEA Inputs"=w1120, "Write ERD List"=w1123, "Error In"=w1119) -> ("GEA Message"=w1125:T3, "Error Out"=w1126:errorcluster)  [unwired: 11 in]
            n83 = call "GEA2MessageFormatter.vi"("Prefix(Send/Recv)"="SEND", "GEA2 Data In"=w1125, "Error In"=w1126) -> ("Output String"=w1127:string, "Error Out"=w1128:errorcluster)  [unwired: 11 in]
            n84 = call "GExplorer_Queue_GEA2.vi"("Output String"=w1127, "error in (no error)"=w1128) -> ("error out"=w1124:errorcluster)  [unwired: 13 in]
            n85 = call "GEA2 Write ERD.vi"("GEA2 Reference In"=w1118, "Read Timeout (ms)"=u32 2000, "GEA Inputs"=w1120, "Write ERD List"=w1123, "Error In"=w1124, "Verify ERD Response?"=FALSE) -> ("GEA2 Reference Out"=w1117:refnum<k24>, "Error Out"=w1116:errorcluster)  [unwired: 7 in, 1 out]
          }
          event "Clear Cycle Buffer": Value Change {
            n86 = event-data() -> ()  [unwired: 1 in, 6 out]
            n87 = Build Array(T24 {"ERD Number"=136, "Data Type"=enum."string", "Data"="FF"} ("ERD Read Data In")) -> (w1143:T24[])
            n88 = call "Convert Write ERD List to Message.vi"("GEA Inputs"=w1138, "Write ERD List"=w1143, "Error In"=w1141) -> ("GEA Message"=w1145:T3, "Error Out"=w1146:errorcluster)  [unwired: 11 in]
            n89 = call "GEA2MessageFormatter.vi"("Prefix(Send/Recv)"="SEND", "GEA2 Data In"=w1145, "Error In"=w1146) -> ("Output String"=w1147:string, "Error Out"=w1148:errorcluster)  [unwired: 11 in]
            n90 = call "GExplorer_Queue_GEA2.vi"("Output String"=w1147, "error in (no error)"=w1148) -> ("error out"=w1144:errorcluster)  [unwired: 13 in]
            n91 = call "GEA2 Write ERD.vi"("GEA2 Reference In"=w1140, "GEA Inputs"=w1138, "Write ERD List"=w1143, "Error In"=w1144) -> ("Error Out"=w1137:errorcluster)  [unwired: 9 in, 2 out]
            n92 = call "Time Delay6"("error in (no error)"=w1137) -> ("error out"=w1132:errorcluster)  [unwired: 10 in]
            n93 = property on="Get Cycle History" class="Bool (strict)"(error in=w1132, "Val(Sgnl)"=TRUE ("Get Cycle History")) -> (error out=w1136:errorcluster)  [unwired: 1 in, 1 out]
            n94 = call "Time Delay7"("error in (no error)"=w1136) -> ("error out"=w1131:errorcluster)  [unwired: 10 in]
            n95 = property on="Get Cycle History" class="Bool (strict)"(error in=w1131, "Val(Sgnl)"=FALSE ("Get Cycle History")) -> (error out=w1135:errorcluster)  [unwired: 1 in, 1 out]
          }
          event "Get Cycle History": Value Change {
            w1155 = T6[] [{"ERD Number"=135, "Data Type"=enum."string"}, {"ERD Number"=57344, "Data Type"=enum."string"}, {"ERD Number"=57345, "Data Type"=enum."string"}, {"ERD Number"=57346, "Data Type"=enum."string"}, {"ERD Number"=57347, "Data Type"=enum."string"}, {"ERD Number"=57348, "Data Type"=enum."string"}, {"ERD Number"=57349, "Data Type"=enum."string"}, {"ERD Number"=57350, "Data Type"=enum."string"}, {"ERD Number"=57351, "Data Type"=enum."string"}, {"ERD Number"=57352, "Data Type"=enum."string"}, {"ERD Number"=57353, "Data Type"=enum."string"}] ("Read ERD List")
            n96 = event-data() -> ()  [unwired: 1 in, 6 out]
            n97 = call "Convert Read ERD List to Message.vi"("GEA Inputs"=w1150, "Read ERD List"=w1155, "Error In"=w1157) -> ("GEA Message"=w1161:T3, "Error Out"=w1162:errorcluster)  [unwired: 11 in]
            n98 = call "GEA2MessageFormatter.vi"("Prefix(Send/Recv)"="SEND", "GEA2 Data In"=w1161, "Error In"=w1162) -> ("Output String"=w1160:string, "Error Out"=w1159:errorcluster)  [unwired: 11 in]
            n99 = call "GExplorer_Queue_GEA2.vi"("Output String"=w1160, "error in (no error)"=w1159) -> ("error out"=w1156:errorcluster)  [unwired: 13 in]
            n100 = call "GEA2 Read ERD Multiple Messages.vi"("GEA2 Reference In"=w1151, "Read Timeout (ms)"=u32 500, "GEA Inputs"=w1150, "Read ERD List"=w1155, "Error In"=w1156, "#ERDs per message"=4, "Verify ERD Response?"=TRUE) -> ("ERD Data Out"=w1163:T30[], "Error Out"=w1154:errorcluster)  [unwired: 5 in, 2 out]
            n101 = call "Cycle_Diag_Table_Read_TL24.vi"("ERD Data In"=w1163, "error in (no error)"=w1154) -> ("Cycle Buffer Status"=→"Cycle Buffer Status":T14, "Diag Cycle String Out"=→"Diagnostics Table":string[][], "error out"=w1149:errorcluster)  [unwired: 10 in, 1 out]
          }
          event "Save Cycle History Log": Value Change {
            w1171 = T6[] [{"ERD Number"=135, "Data Type"=enum."string"}, {"ERD Number"=57344, "Data Type"=enum."string"}, {"ERD Number"=57345, "Data Type"=enum."string"}, {"ERD Number"=57346, "Data Type"=enum."string"}, {"ERD Number"=57347, "Data Type"=enum."string"}, {"ERD Number"=57348, "Data Type"=enum."string"}, {"ERD Number"=57349, "Data Type"=enum."string"}, {"ERD Number"=57350, "Data Type"=enum."string"}, {"ERD Number"=57351, "Data Type"=enum."string"}, {"ERD Number"=57352, "Data Type"=enum."string"}, {"ERD Number"=57353, "Data Type"=enum."string"}] ("Read ERD List")
            n102 = event-data() -> ()  [unwired: 1 in, 6 out]
            n103 = call "Convert Read ERD List to Message.vi"("GEA Inputs"=w1174, "Read ERD List"=w1171, "Error In"=w1173) -> ("GEA Message"=w1180:T3, "Error Out"=w1181:errorcluster)  [unwired: 11 in]
            n104 = call "GEA2MessageFormatter.vi"("Prefix(Send/Recv)"="SEND", "GEA2 Data In"=w1180, "Error In"=w1181) -> ("Output String"=w1179:string, "Error Out"=w1178:errorcluster)  [unwired: 11 in]
            n105 = call "GExplorer_Queue_GEA2.vi"("Output String"=w1179, "error in (no error)"=w1178) -> ("error out"=w1176:errorcluster)  [unwired: 13 in]
            n106 = call "GEA2 Read ERD Multiple Messages.vi"("GEA2 Reference In"=w1172, "Read Timeout (ms)"=u32 500, "GEA Inputs"=w1174, "Read ERD List"=w1171, "Error In"=w1176, "#ERDs per message"=4, "Verify ERD Response?"=TRUE) -> ("ERD Data Out"=w1170:T30[], "Error Out"=w1175:errorcluster)  [unwired: 5 in, 2 out]
            n107 = call "Cycle_Diag_Table_Read_TL24.vi"("ERD Data In"=w1170, "error in (no error)"=w1175) -> ("Diag Cycle String Out"=w1169:string[][], "error out"=w1168:errorcluster)  [unwired: 10 in, 2 out]
            n108 = call "Cycle_History_Logging.vi"("error in (no error)"=w1168, "Diag Cycle String Out"=w1169) -> ("error out"=w1167:errorcluster)  [unwired: 9 in]
          }
          event "Data ON": Value Change {
            n109 = event-data() -> ()  [unwired: 1 in, 6 out]
            n110 = case shown="True" "Data ON" {
              tunnel: w1188 -> [w1191 w1195]
              tunnel: [w1190 w1194] -> w1187
              tunnel: w1185 -> [w1189 w1193]
              frame True {
                n111 = Enqueue Element(queue=w1189, element=T21 {"Data"=variant, "State"=enum."Init"} ("Data"), error in (no error)=w1191) -> (error out=w1190:errorcluster)  [unwired: 1 in, 2 out]
              }
              frame False {
                n112 = Enqueue Element(queue=w1193, element=T21 {"Data"=variant, "State"=enum."Pause"} ("Data"), error in (no error)=w1195) -> (error out=w1194:errorcluster)  [unwired: 1 in, 2 out]
              }
            }
          }
          event "Stop": Value Change; User Event; Panel Close {
            n113 = event-data() -> ()  [unwired: 1 in, 3 out]
            n114 = call "Control_ERD_Loop_Brass.vi"("Command (ERD Loop Control)"=ERD_Loop_Control_Command_Brass."Shutdown", "Error In"=w1205) -> ("Error Out"=w1204:errorcluster)  [unwired: 13 in]
            n115 = call "Control_GEA2_Loop_Brass.vi"("Command (ERD Loop Control)"=GEA2_Control_Command_Brass."Shutdown", "Error In"=w1204) -> ("Error Out"=w1206:errorcluster)  [unwired: 13 in]
            n116 = call "Control_DAQ_Loop_Brass.vi"("Command (DAQ Control)"=DAQ_Control_Command_Brass."Shutdown", "Error In"=w1206) -> ("Error Out"=w1209:errorcluster)  [unwired: 13 in]
            n117 = call "Control_Cont_Send_Brass.vi"("Command (ERD Loop Control)"=GEA2_Control_Command_Brass."Shutdown", "Error In"=w1209) -> ("Error Out"=w1199:errorcluster)  [unwired: 13 in]
            n118 = call "Time Delay8"("error in (no error)"=w1199, "Delay Time (s)"=2.0) -> ("error out"=w1198:errorcluster)  [unwired: 9 in]
          }
        }
        n119 = call "Error_Control_Brass.vi"("Error In"=w1006) -> ("Error Out"=w1008:errorcluster)  [unwired: 14 in]
      }
      n120 = Unbundle By Name(T21 {"Data"=variant, "State"=enum."Init"} ("Data")) -> ("State"=w67:T22)
      n121 = Build Array(w62, w60, w61) -> (w59:refnum<vi>[])
      n122 = while "DAQ Loop" {
        shift-right: [w481] -> w94
        shift-left: w31 -> [w479]
        shift-right: [w458] -> _
        shift-left: DAQ_States_Brass."Wait for Init" ("States") -> [w476]
        shift-right: [w459] -> _
        shift-left: "Wait for Init" ("Report Text") -> [w474]
        tunnel: w58 -> [w475]
        shift-right: [w457] -> _
        shift-left: _ -> [w414]
        shift-right: [w456] -> _
        shift-left: FALSE -> [w455]
        shift-right: [w445] -> _
        shift-left: w50 -> [w444]
        shift-right: [w443] -> _
        shift-left: w50 -> [w442]
        shift-right: [w441] -> _
        shift-left: w50 -> [w440]
        shift-right: [w439] -> _
        shift-left: w50 -> [w438]
        shift-right: [w437] -> _
        shift-left: w50 -> [w436]
        shift-right: [w435] -> _
        shift-left: w50 -> [w434]
        shift-right: [w433] -> _
        shift-left: w50 -> [w432]
        shift-right: [w419] -> _
        shift-left: 1.0 -> [w415]
        shift-right: [w418] -> _
        shift-left: 1.0 -> [w422]
        shift-right: [w417] -> _
        shift-left: 0.0 -> [w421]
        shift-right: [w413] -> _
        shift-left: w50 -> [w412]
        shift-right: [w411] -> _
        shift-left: FALSE -> [w446]
        stop <- w471 stop-if-true
        # "Automatic Modeshift Feedback"
        # "DAQ Loop"
        n123 = Greater?(x=w422, y=5.0 ("x")) -> (0:w424:bool)
        n124 = Dequeue Element(queue=w475, timeout in ms (-1)=0, error in (no error)=w479) -> (element=w477:T20, timed out?=w478:bool, error out=w470:errorcluster)  [unwired: 1 out]
        n125 = Wait (ms)(milliseconds to wait=u32 250) -> ()  [unwired: 1 out]
        n126 = Select(t="Basket RPM", s=w424, f=w415) -> (s? t:f=w419:dbl)
        n127 = Select(t=w476, s=w478, f=w477) -> (s? t:f=w473:T20)
        n128 = Multiply(x=w419, y=0.40625) -> (x*y=w450:dbl)
        n129 = Less?(x=w419, y=1.0) -> (x < y?=w448:bool)
        n130 = Equal?(x=w415, y=w419) -> (x = y?=w447:bool)
        n131 = case shown="\"Run\"" w473 {
          selector: w473 -> [_ _ _ _ _ _ w960]
          tunnel: [_ _ _ w673 w793 _ _] -> w413
          tunnel: [w513 w537 w569 w674 w791 w898 w963] -> w467
          tunnel: w432 -> [w528 w552 w577 _ w790 w892 w909]
          tunnel: [w528 w552 w577 w678 w789 _ _] -> w433
          tunnel: w434 -> [w527 w551 w578 _ w788 w889 w936]
          tunnel: [w527 w551 w578 w682 w787 _ _] -> w435
          tunnel: [w511 w535 w561 w681 w786 w852 w926] -> w465
          tunnel: [w512 w536 w562 w677 w785 w859 w938] -> w466
          tunnel: [w522 DAQ_States_Brass."Verify Hardware" ("t") w574 DAQ_States_Brass."Run" ("t") w763 DAQ_States_Brass."Wait for Init" ("States") w960] -> w458
          tunnel: [FALSE FALSE FALSE TRUE TRUE FALSE FALSE] -> w457
          tunnel: w440 -> [w526 w550 w581 _ w748 w896 w965]
          tunnel: [w508 w532 w558 w670 w782 w845 w923] -> w462
          tunnel: [w526 w550 w581 w671 w783 _ _] -> w441
          tunnel: [w509 w533 w559 w634 w773 w884 w964] -> w463
          tunnel: w438 -> [w525 w549 w580 _ w772 w895 w959]
          tunnel: [w525 w549 w580 w639 w774 _ _] -> w439
          tunnel: [_ _ _ _ _ FALSE TRUE] -> w471
          tunnel: [_ _ _ _ w781 _ _] -> w431
          tunnel: [_ _ _ _ w775 _ _] -> w416
          tunnel: [_ _ _ _ w780 _ _] -> w430
          tunnel: [_ _ _ _ w779 _ _] -> w429
          tunnel: [_ _ _ _ w778 _ _] -> w428
          tunnel: [_ _ _ _ w777 _ _] -> w427
          tunnel: [_ _ _ _ w776 _ _] -> w426
          tunnel: [w510 w534 w560 w631 w771 w882 w957] -> w464
          tunnel: [w524 w548 w579 w628 w769 _ _] -> w437
          tunnel: w436 -> [w524 w548 w579 _ w770 w883 w958]
          tunnel: [_ _ _ _ w768 _ _] -> w454
          tunnel: [_ _ _ _ w767 _ _] -> w453
          tunnel: [w523 w547 w571 "Initialize" ("Report Text") "Running" ("Report Text") "Wait for Init" ("Report Text") "Exit" ("Report Text")] -> w459
          tunnel: w474 -> [w523 w547 _ _ _ _ _]
          tunnel: [w507 w531 w557 w612 w755 w876 w954] -> w461
          tunnel: [w518 w545 w567 w609 w754 _ _] -> w443
          tunnel: [w517 w544 w566 w607 w752 _ _] -> w445
          tunnel: [w506 w530 w556 w606 w753 w875 w901] -> w460
          tunnel: w442 -> [w518 w545 w567 _ w756 w877 w955]
          tunnel: w444 -> [w517 w544 w566 _ w751 w873 w921]
          tunnel: [w505 w529 w555 w586 w750 FALSE FALSE] -> w456
          tunnel: [FALSE FALSE FALSE FALSE w740 FALSE FALSE] -> w411
          tunnel: [w514 w540 w564 w593 w739 w868 w951] -> w468
          tunnel: "Turn On DAQ" -> [w515 _ _ _ w715 _ _]
          tunnel: w470 -> [w513 w537 w563 w595 w738 w867 w950]
          tunnel: w470 -> [w512 w536 w562 w594 w733 w865 w912]
          tunnel: w470 -> [w514 w539 w564 w593 w739 w868 w951]
          tunnel: w470 -> [w511 w535 w561 w592 w731 w850 w935]
          tunnel: w470 -> [w510 w534 w560 w591 w730 w849 w949]
          tunnel: w470 -> [w509 w533 w559 w590 w727 w848 w948]
          tunnel: w470 -> [w508 w532 w558 w589 w726 w847 w947]
          tunnel: w470 -> [w507 w531 w557 w588 w720 w843 w946]
          tunnel: w470 -> [w506 w530 w556 w587 w716 w842 w920]
          tunnel: w455 -> [w505 w529 w555 w586 w719 _ _]
          tunnel: w450 -> [_ _ _ _ w725 _ _]
          tunnel: 0.5 ("Duty Cycle") -> [_ _ _ _ w724 _ _]
          tunnel: w448 -> [_ _ _ _ w722 _ _]
          tunnel: w447 -> [_ _ _ _ w723 _ _]
          tunnel: w446 -> [_ _ _ _ w721 _ _]
          tunnel: w414 -> [_ _ _ _ _ _ w945]
          tunnel: w412 -> [_ _ _ _ w714 w841 w944]
          frame "Wait for Init", Default {
            # "Hall Sensor"
            # "Motor TRIAC CCW"
            # "Motor TRIAC CW"
            # "Relay Controls"
            # "TRIAC Outputs"
            # "AO for ADC"
            n132 = Select(t=DAQ_States_Brass."Rename Devices", s=w515, f=DAQ_States_Brass."Wait for Init" ("States")) -> (s? t:f=w522:T20)
          }
          frame "Rename Devices" {
            # "Hall Sensor"
            # "Motor TRIAC CCW"
            # "Motor TRIAC CW"
            # "Relay Controls"
            # "TRIAC Outputs"
            n133 = case shown="\"LE\"" "HE/LE ?" {
              tunnel: ["VALEW_HE" "VALEW_LE"] -> w541
              frame "HE", Default {
              }
              frame "LE" {
              }
            }
            n134 = call "VALEW_Rename DAQmx Devices.vi"("cDAQ Name"=w541, "Error In"=w539) -> ("Error Out"=w540:errorcluster)  [unwired: 13 in]
          }
          frame "Verify Hardware" {
            n135 = call "DeviceListCheck.vi"("Device List"=string[] ["9481_1", "9435_1", "9435_2", "9401_1", "9269_1"], "Error In"=w563) -> ("Devices Present?"=w568:bool, "Report Text"=w571:string, "Error Out"=w570:errorcluster)  [unwired: 11 in]
            n136 = case shown="False" w568 {
              selector: w568 -> [w583 _]
              tunnel: w570 -> [w584 w585]
              tunnel: [w582 w585] -> w569
              frame False {
                n137 = property on="Turn On DAQ" class="Bool (strict)"(error in=w584, "Value"=w583) -> (error out=w582:errorcluster)  [unwired: 1 in, 1 out]
              }
              frame True {
              }
            }
            n138 = Select(t=DAQ_States_Brass."Initialize" ("f"), s=w568, f=DAQ_States_Brass."Wait for Init") -> (s? t:f=w574:T20)
          }
          frame "Initialize" {
            w600 = 4 items=["verify"=2, "reserve"=4, "commit"=3, "unreserve"=5, "abort"=6] ("action")
            w616 = 10123 items=["Finite Samples"=10178, "Continuous Samples"=10123, "Hardware Timed Single Point"=12522] ("sample mode")
            w619 = 4 items=["verify"=2, "reserve"=4, "commit"=3, "unreserve"=5, "abort"=6] ("action")
            w652 = 4 items=["verify"=2, "reserve"=4, "commit"=3, "unreserve"=5, "abort"=6] ("action")
            w653 = 4 items=["verify"=2, "reserve"=4, "commit"=3, "unreserve"=5, "abort"=6] ("action")
            w667 = 10123 items=["Finite Samples"=10178, "Continuous Samples"=10123, "Hardware Timed Single Point"=12522] ("sample mode")
            w675 = 0 items=["one channel for each line", "one channel for all lines"] ("line grouping")
            w680 = 0 items=["one channel for each line", "one channel for all lines"] ("line grouping")
            w683 = 0.0  # minimum value
            w684 = 5.0  # maximum value
            # "Hall Sensor"
            # "Motor TRIAC CCW"
            # "Motor TRIAC CW"
            # "Relay Controls"
            # "TRIAC Outputs"
            # "AO for ADC"
            n139 = call <vilib>:"DAQmx Create Task.vi"("auto cleanup"=TRUE, "error in"=w589) -> ("task out"=w641:refnum<k21>, "error out"=w642:errorcluster)  [unwired: 12 in]
            n140 = call <vilib>:"DAQmx Create Task.vi"("auto cleanup"=TRUE, "error in"=w588) -> ("task out"=w615:refnum<k21>, "error out"=w614:errorcluster)  [unwired: 12 in]
            n141 = call <vilib>:"DAQmx Create Task.vi"("auto cleanup"=TRUE, "error in"=w591) -> ("task out"=w649:refnum<k21>, "error out"=w650:errorcluster)  [unwired: 12 in]
            n142 = call <vilib>:"DAQmx Create Task.vi"("auto cleanup"=TRUE, "error in"=w590) -> ("task out"=w647:refnum<k21>, "error out"=w648:errorcluster)  [unwired: 12 in]
            n143 = call-poly <vilib>:"DAQmx Create Virtual Channel.vi"("task in"=w641, "counter"=tag "9401_1/ctr2", "error in"=w642) -> ("task out"=w644:refnum<k21>, "error out"=w672:errorcluster)  [unwired: 11 in]
            n144 = call-poly <vilib>:"DAQmx Create Virtual Channel.vi"("task in"=w649, "counter"=tag "9401_1/ctr0", "error in"=w650) -> ("task out"=w662:refnum<k21>, "error out"=w658:errorcluster)  [unwired: 11 in]
            n145 = call-poly <vilib>:"DAQmx Create Virtual Channel.vi"("task in"=w647, "counter"=tag "9401_1/ctr1", "error in"=w648) -> ("task out"=w661:refnum<k21>, "error out"=w660:errorcluster)  [unwired: 11 in]
            n146 = call-poly <vilib>:"DAQmx Create Virtual Channel.vi"("task in"=w615, "lines"=tag "9401_1/port0/line2", "error in"=w614) -> ("task out"=w621:refnum<k21>, "error out"=w622:errorcluster)  [unwired: 11 in]
            n147 = property class="DAQmx Channel"(reference=w644, error in=w672, "CO.Pulse.Term"=tag "/9401_1/PFI4") -> (reference out=w669:refnum<k21>, error out=w668:errorcluster)
            n148 = call-poly <vilib>:"DAQmx Create Virtual Channel.vi"("lines"=tag "9481_1/port0/line3", "error in"=w587) -> ("task out"=w607:refnum<k21>, "error out"=w606:errorcluster)  [unwired: 12 in]
            n149 = property class="DAQmx Channel"(reference=w662, error in=w658, "CI.CountEdges.Term"=tag "/9401_1/PFI0") -> (reference out=w657:refnum<k21>, error out=w656:errorcluster)
            n150 = property class="DAQmx Channel"(reference=w661, error in=w660, "CI.CountEdges.Term"=tag "/9401_1/PFI1") -> (reference out=w655:refnum<k21>, error out=w654:errorcluster)
            n151 = call-poly <vilib>:"DAQmx Create Virtual Channel.vi"("lines"=tag "9481_1/port0/line0:2", "name to assign"="Relay Outputs", "line grouping"=w680, "error in"=w594) -> ("task out"=w678:refnum<k21>, "error out"=w677:errorcluster)  [unwired: 10 in]
            n152 = call-poly <vilib>:"DAQmx Create Virtual Channel.vi"("lines"=tag "9435_1/port0/line0:2, 9435_2/port0/line0:3", "name to assign"="Outputs", "line grouping"=w675, "error in"=w595) -> ("task out"=w673:refnum<k21>, "error out"=w674:errorcluster)  [unwired: 10 in]
            n153 = call-poly <vilib>:"DAQmx Create Virtual Channel.vi"("maximum value"=w684, "minimum value"=w683, "physical channels"=tag "9269_1/ao0:2" ("lines"), "name to assign"="AO for ADC", "error in"=w592) -> ("task out"=w682:refnum<k21>, "error out"=w681:errorcluster)  [unwired: 9 in]
            n154 = call-poly <vilib>:"DAQmx Timing.vi"("task/channels in"=w621, "sample mode"=w616, "rate"=1000.0, "error in"=w622) -> ("task out"=w617:refnum<k21>, "error out"=w618:errorcluster)  [unwired: 10 in]
            n155 = call-poly <vilib>:"DAQmx Timing.vi"("task/channels in"=w669, "sample mode"=w667, "error in"=w668) -> ("task out"=w599:refnum<k21>, "error out"=w596:errorcluster)  [unwired: 11 in]
            n156 = call <vilib>:"DAQmx Control Task.vi"("task/channels in"=w657, "action"=w652, "error in"=w656) -> ("task out"=w630:refnum<k21>, "error out"=w633:errorcluster)  [unwired: 11 in]
            n157 = call <vilib>:"DAQmx Control Task.vi"("task/channels in"=w655, "action"=w653, "error in"=w654) -> ("task out"=w638:refnum<k21>, "error out"=w636:errorcluster)  [unwired: 11 in]
            n158 = call <vilib>:"DAQmx Control Task.vi"("task/channels in"=w599, "action"=w600, "error in"=w596) -> ("task out"=w598:refnum<k21>, "error out"=w597:errorcluster)  [unwired: 11 in]
            n159 = call <vilib>:"DAQmx Control Task.vi"("task/channels in"=w617, "action"=w619, "error in"=w618) -> ("task out"=w610:refnum<k21>, "error out"=w611:errorcluster)  [unwired: 11 in]
            n160 = flat-sequence {
              tunnel: w598 -> [w688]
              tunnel: w597 -> [w687]
              tunnel: w638 -> [w696]
              tunnel: [w696] -> w637
              tunnel: w636 -> [w695]
              tunnel: [w695] -> w635
              tunnel: w633 -> [w694]
              tunnel: [w694] -> w632
              tunnel: w630 -> [w693]
              tunnel: [w693] -> w629
              tunnel: w611 -> [w691]
              tunnel: w610 -> [w692]
              tunnel: [w690] -> w604
              tunnel: [w689] -> w603
              tunnel: [w688] -> w602
              tunnel: [w687] -> w601
              tunnel: [w700] -> w670
              tunnel: [w699] -> w671
              tunnel: [w710] -> w639
              tunnel: w637 -> [w709]
              tunnel: w635 -> [w708]
              tunnel: [w707] -> w634
              tunnel: w632 -> [w706]
              tunnel: [w705] -> w631
              tunnel: w629 -> [w704]
              tunnel: [w703] -> w628
              tunnel: [w702] -> w612
              tunnel: [w701] -> w609
              tunnel: w604 -> [w702]
              tunnel: w603 -> [w701]
              tunnel: w602 -> [w698]
              tunnel: w601 -> [w697]
              frame #0 {
                n161 = call <vilib>:"DAQmx Start Task.vi"("task/channels in"=w692, "error in"=w691) -> ("task out"=w689:refnum<k21>, "error out"=w690:errorcluster)  [unwired: 12 in]
              }
              frame #1 {
                n162 = call <vilib>:"DAQmx Start Task.vi"("task/channels in"=w704, "error in"=w706) -> ("task out"=w703:refnum<k21>, "error out"=w705:errorcluster)  [unwired: 12 in]
                n163 = call <vilib>:"DAQmx Start Task.vi"("task/channels in"=w709, "error in"=w708) -> ("task out"=w710:refnum<k21>, "error out"=w707:errorcluster)  [unwired: 12 in]
                n164 = call <vilib>:"DAQmx Start Task.vi"("task/channels in"=w698, "error in"=w697) -> ("task out"=w699:refnum<k21>, "error out"=w700:errorcluster)  [unwired: 12 in]
              }
            }
          }
          frame "Run" {
            # "Lid Lock Feedback"
            # "Is the task stopped?"
            # "Hall Sensor"
            # "Motor TRIAC CCW"
            # "Motor TRIAC CW"
            # "AO for ADC"
            # "Relay Controls"
            # "TRIAC Outputs"
            n165 = case shown="True" w722 {
              tunnel: w748 -> [w827 w832]
              tunnel: [w827 w831] -> w746
              tunnel: [w826 w830] -> w747
              tunnel: [w825 TRUE] -> w741
              tunnel: w726 -> [w826 w828]
              tunnel: w721 -> [w825 _]
              frame False {
              }
              frame True {
                n166 = call <vilib>:"DAQmx Stop Task.vi"("task/channels in"=w832, "error in"=w828) -> ("task out"=w831:refnum<k21>, "error out"=w830:errorcluster)  [unwired: 12 in]
              }
            }
            n167 = call-poly <vilib>:"DAQmx Read.vi"("task/channels in"=w756, "number of samples per channel"=-1, "timeout"=10.0, "error in"=w720) -> ("task out"=w754:refnum<k21>, "data"=w760:u8[], "error out"=w755:errorcluster)  [unwired: 9 in]
            n168 = Compound Arithmetic op=AND(w741, invert w722) -> (w743:bool)
            n169 = case shown="False" w743 {
              tunnel: w747 -> [w817 w821]
              tunnel: w746 -> [w818 w820]
              tunnel: [w818 w824] -> w745
              tunnel: [w817 w823] -> w744
              tunnel: w741 -> [w816 _]
              tunnel: [w816 FALSE] -> w740
              frame False {
              }
              frame True {
                n170 = call <vilib>:"DAQmx Start Task.vi"("task/channels in"=w820, "error in"=w821) -> ("task out"=w824:refnum<k21>, "error out"=w823:errorcluster)  [unwired: 12 in]
                n171 = Wait (ms)(milliseconds to wait=u32 1200) -> ()  [unwired: 1 out]
              }
            }
            n172 = Build Array("AC Power", "Mode Shift FB", "Lid Status") -> (w734:bool[])
            n173 = Build Array("Pressure", "Motor Current", "Temperature") -> (w732:dbl[])
            n174 = Search 1D Array(1D array=w760, element=u8 4) -> (index of element=w758:i32)  [unwired: 1 in]
            n175 = Equal?(x=w758, y=-1) -> (x = y?=w749:bool)
            n176 = Compound Arithmetic op=OR(w722, w723) -> (w742:bool)
            n177 = call-poly <vilib>:"DAQmx Read.vi"("task/channels in"=w714, "error in"=w738) -> ("task out"=w793:refnum<k21>, "data"=w792:bool[], "error out"=w791:errorcluster)  [unwired: 11 in]
            n178 = call-poly <vilib>:"DAQmx Write.vi"("task/channels in"=w790, "data"=w734, "error in"=w733) -> ("task out"=w789:refnum<k21>, "error out"=w785:errorcluster)  [unwired: 10 in, 1 out]
            n179 = call-poly <vilib>:"DAQmx Write.vi"("task/channels in"=w788, "data"=w732, "error in"=w731) -> ("task out"=w787:refnum<k21>, "error out"=w786:errorcluster)  [unwired: 10 in, 1 out]
            n180 = call-poly <vilib>:"DAQmx Read.vi"("task/channels in"=w770, "error in"=w730) -> ("task out"=w769:refnum<k21>, "data"=w729:u32, "error out"=w771:errorcluster)  [unwired: 11 in]
            "CW" <- w729
            n181 = call-poly <vilib>:"DAQmx Read.vi"("task/channels in"=w772, "error in"=w727) -> ("task out"=w774:refnum<k21>, "data"=w728:u32, "error out"=w773:errorcluster)  [unwired: 11 in]
            "CCW" <- w728
            n182 = case shown="True" "LL (M - A)" {
              tunnel: [w796 w806] -> w753
              tunnel: [w797 w805] -> w752
              tunnel: w751 -> [w799 w804]
              tunnel: [w795 w803] -> w750
              tunnel: w749 -> [_ w802]
              tunnel: "Lid Lock Feedback" -> [w798 _]
              tunnel: w719 -> [w795 w801]
              tunnel: w716 -> [w794 w800]
              frame False {
                n183 = call-poly <vilib>:"DAQmx Write.vi"("task/channels in"=w799, "data"=w798, "error in"=w794) -> ("task out"=w797:refnum<k21>, "error out"=w796:errorcluster)  [unwired: 10 in, 1 out]
              }
              frame True {
                # "Automatic Lid Lock feedback"
                n184 = case shown="True" w802 {
                  tunnel: w804 -> [w812 w815]
                  tunnel: [w811 w814] -> w806
                  tunnel: [w810 w815] -> w805
                  tunnel: [w809 w813] -> w803
                  tunnel: w801 -> [w808 w813]
                  tunnel: w800 -> [w807 w814]
                  frame False {
                    n185 = Not(x=w808) -> (.not. x?=w809:bool)
                    n186 = call-poly <vilib>:"DAQmx Write.vi"("task/channels in"=w812, "data"=w809, "error in"=w807) -> ("task out"=w810:refnum<k21>, "error out"=w811:errorcluster)  [unwired: 10 in, 1 out]
                  }
                  frame True {
                  }
                }
              }
            }
            n187 = Index Array(array=w792) -> (element #1=w781:bool, element #2=w775:bool, element #3=w780:bool, element #4=w779:bool, element #5=w778:bool, element #6=w777:bool, element #7=w776:bool)  [unwired: 7 in]
            n188 = call "Counts to Triac Direction.vi"("CCW ctr"=w728, "CW ctr"=w729) -> ("CW"=w767:bool, "CCW"=w768:bool)  [unwired: 8 in]
            n189 = case shown="False" w742 {
              tunnel: w745 -> [w838 w840]
              tunnel: w744 -> [w837 w839]
              tunnel: [w836 w840] -> w783
              tunnel: [w835 w839] -> w782
              tunnel: w725 -> [w834 _]
              tunnel: w724 -> [w833 _]
              frame False {
                n190 = property class="DAQmx Channel"(reference=w838, error in=w837, "CO.Pulse.Freq"=w834, "CO.Pulse.DutyCyc"=w833) -> (reference out=w836:refnum<k21>, error out=w835:errorcluster)
              }
              frame True {
              }
            }
            n191 = Select(t=DAQ_States_Brass."Run" ("States"), s=w715, f=DAQ_States_Brass."Shutdown" ("States")) -> (s? t:f=w763:T20)
          }
          frame "Shutdown" {
            w881 = 0.0
            w878 = FALSE ("element")
            # "Hall Sensor"
            # "Motor TRIAC CCW"
            # "Motor TRIAC CW"
            # "Relay Controls"
            # "TRIAC Outputs"
            # "AO for ADC"
            n192 = local read "AC Power"() -> (w866:bool)
            n193 = Build Array(w866, w878, w878) -> (w893:bool[])
            n194 = Build Array(w881, w881, w881) -> (w880:dbl[])
            n195 = call-poly <vilib>:"DAQmx Write.vi"("task/channels in"=w892, "data"=w893, "error in"=w865) -> ("task out"=w886:refnum<k21>, "error out"=w887:errorcluster)  [unwired: 10 in, 1 out]
            n196 = call-poly <vilib>:"DAQmx Write.vi"("task/channels in"=w873, "data"=FALSE, "error in"=w842) -> ("task out"=w872:refnum<k21>, "error out"=w871:errorcluster)  [unwired: 10 in, 1 out]
            n197 = call-poly <vilib>:"DAQmx Write.vi"("task/channels in"=w889, "data"=w880, "error in"=w850) -> ("task out"=w891:refnum<k21>, "error out"=w890:errorcluster)  [unwired: 10 in, 1 out]
            n198 = call "Time Delay4"("error in (no error)"=w887, "Delay Time (s)"=2.0) -> ("error out"=w885:errorcluster)  [unwired: 9 in]
            n199 = call <vilib>:"DAQmx Clear Task.vi"("task in"=w877, "error in"=w843) -> ("error out"=w876:errorcluster)  [unwired: 13 in]
            n200 = call <vilib>:"DAQmx Clear Task.vi"("task in"=w841, "error in"=w867) -> ("error out"=w898:errorcluster)  [unwired: 13 in]
            n201 = call <vilib>:"DAQmx Clear Task.vi"("task in"=w886, "error in"=w885) -> ("error out"=w864:errorcluster)  [unwired: 13 in]
            n202 = call <vilib>:"DAQmx Clear Task.vi"("task in"=w891, "error in"=w890) -> ("error out"=w857:errorcluster)  [unwired: 13 in]
            n203 = call <vilib>:"DAQmx Clear Task.vi"("task in"=w883, "error in"=w849) -> ("error out"=w882:errorcluster)  [unwired: 13 in]
            n204 = call <vilib>:"DAQmx Clear Task.vi"("task in"=w895, "error in"=w848) -> ("error out"=w884:errorcluster)  [unwired: 13 in]
            n205 = call <vilib>:"DAQmx Clear Task.vi"("task in"=w896, "error in"=w847) -> ("error out"=w846:errorcluster)  [unwired: 13 in]
            n206 = call <vilib>:"DAQmx Clear Task.vi"("task in"=w872, "error in"=w871) -> ("error out"=w875:errorcluster)  [unwired: 13 in]
            n207 = property on="Motor Current" class="Slide (strict)"(error in=w857, "Value"=2.5 ("Motor Current")) -> (error out=w855:errorcluster)  [unwired: 1 in, 1 out]
            n208 = property on="Turn On DAQ" class="Bool (strict)"(error in=w864, "Value"=FALSE ("Turn On DAQ")) -> (error out=w862:errorcluster)  [unwired: 1 in, 1 out]
            n209 = property on="Basket RPM" class="DigNum (strict)"(error in=w846, "Value"=1.0 ("Basket RPM")) -> (error out=w845:errorcluster)  [unwired: 1 in, 1 out]
            n210 = property on="Temperature" class="Slide (strict)"(error in=w855, "Value"=2.5 ("Temperature")) -> (error out=w853:errorcluster)  [unwired: 1 in, 1 out]
            n211 = property on="Mode Shift FB" class="Bool (strict)"(error in=w862, "Value"=FALSE ("Mode Shift FB")) -> (error out=w860:errorcluster)  [unwired: 1 in, 1 out]
            n212 = property on="Lid Status" class="Bool (strict)"(error in=w860, "Value"=FALSE ("Lid Status")) -> (error out=w859:errorcluster)  [unwired: 1 in, 1 out]
            n213 = property on="Pressure" class="Slide (strict)"(error in=w853, "Value"=0.0 ("Pressure")) -> (error out=w852:errorcluster)  [unwired: 1 in, 1 out]
          }
          frame "Exit" {
            w916 = FALSE ("element")
            w934 = 0.0
            n214 = local read "AC Power"() -> (w917:bool)
            n215 = Build Array(w917, w916, w916) -> (w913:bool[])
            n216 = call-poly <vilib>:"DAQmx Write.vi"("task/channels in"=w909, "data"=w913, "error in"=w912) -> ("task out"=w910:refnum<k21>, "error out"=w915:errorcluster)  [unwired: 10 in, 1 out]
            n217 = Build Array(w934, w934, w934) -> (w937:dbl[])
            n218 = call-poly <vilib>:"DAQmx Write.vi"("task/channels in"=w921, "data"=FALSE, "error in"=w920) -> ("task out"=w919:refnum<k21>, "error out"=w918:errorcluster)  [unwired: 10 in, 1 out]
            n219 = call-poly <vilib>:"DAQmx Write.vi"("task/channels in"=w936, "data"=w937, "error in"=w935) -> ("task out"=w933:refnum<k21>, "error out"=w932:errorcluster)  [unwired: 10 in, 1 out]
            n220 = call "Time Delay"("error in (no error)"=w915, "Delay Time (s)"=2.0) -> ("error out"=w911:errorcluster)  [unwired: 9 in]
            n221 = case shown="True" w945 {
              tunnel: w910 -> [_ w997]
              tunnel: w965 -> [_ w996]
              tunnel: [w969 w995] -> w924
              tunnel: [w970 w994] -> w964
              tunnel: [w966 w993] -> w904
              tunnel: [w972 w992] -> w907
              tunnel: [w973 w991] -> w963
              tunnel: w959 -> [_ w990]
              tunnel: w958 -> [_ w989]
              tunnel: [w971 w988] -> w957
              tunnel: w955 -> [_ w987]
              tunnel: [w968 w986] -> w954
              tunnel: w919 -> [_ w985]
              tunnel: [w967 w984] -> w902
              tunnel: w950 -> [w973 w983]
              tunnel: w911 -> [w972 w982]
              tunnel: w949 -> [w971 w981]
              tunnel: w948 -> [w970 w980]
              tunnel: w947 -> [w969 w979]
              tunnel: w946 -> [w968 w978]
              tunnel: w918 -> [w967 w977]
              tunnel: w944 -> [_ w976]
              tunnel: w933 -> [_ w975]
              tunnel: w932 -> [w966 w974]
              frame False {
              }
              frame True {
                # "Hall Sensor"
                # "Motor TRIAC CCW"
                # "Motor TRIAC CW"
                # "Relay Controls"
                # "TRIAC Outputs"
                # "AO for ADC"
                n222 = call <vilib>:"DAQmx Clear Task.vi"("task in"=w987, "error in"=w978) -> ("error out"=w986:errorcluster)  [unwired: 13 in]
                n223 = call <vilib>:"DAQmx Clear Task.vi"("task in"=w985, "error in"=w977) -> ("error out"=w984:errorcluster)  [unwired: 13 in]
                n224 = call <vilib>:"DAQmx Clear Task.vi"("task in"=w976, "error in"=w983) -> ("error out"=w991:errorcluster)  [unwired: 13 in]
                n225 = call <vilib>:"DAQmx Clear Task.vi"("task in"=w997, "error in"=w982) -> ("error out"=w992:errorcluster)  [unwired: 13 in]
                n226 = call <vilib>:"DAQmx Clear Task.vi"("task in"=w975, "error in"=w974) -> ("error out"=w993:errorcluster)  [unwired: 13 in]
                n227 = call <vilib>:"DAQmx Clear Task.vi"("task in"=w989, "error in"=w981) -> ("error out"=w988:errorcluster)  [unwired: 13 in]
                n228 = call <vilib>:"DAQmx Clear Task.vi"("task in"=w990, "error in"=w980) -> ("error out"=w994:errorcluster)  [unwired: 13 in]
                n229 = call <vilib>:"DAQmx Clear Task.vi"("task in"=w996, "error in"=w979) -> ("error out"=w995:errorcluster)  [unwired: 13 in]
              }
            }
            n230 = call <vilib>:"Clear Errors.vi"("error in (no error)"=w904, "specific error code to clear (0: all)"=-200088) -> ("error out"=w903:errorcluster)  [unwired: 4 in, 1 out]
            n231 = call <vilib>:"Clear Errors.vi"("error in (no error)"=w907, "specific error code to clear (0: all)"=-200088) -> ("error out"=w906:errorcluster)  [unwired: 4 in, 1 out]
            n232 = call <vilib>:"Clear Errors.vi"("error in (no error)"=w902, "specific error code to clear (0: all)"=-200088) -> ("error out"=w901:errorcluster)  [unwired: 4 in, 1 out]
            n233 = property on="Turn On DAQ" class="Bool (strict)"(error in=w906, "Value"=FALSE ("Turn On DAQ")) -> (error out=w942:errorcluster)  [unwired: 1 in, 1 out]
            n234 = property on="Motor Current" class="Slide (strict)"(error in=w903, "Value"=2.5 ("Motor Current")) -> (error out=w930:errorcluster)  [unwired: 1 in, 1 out]
            n235 = property on="Basket RPM" class="DigNum (strict)"(error in=w924, "Value"=1.0 ("Basket RPM")) -> (error out=w923:errorcluster)  [unwired: 1 in, 1 out]
            n236 = property on="Mode Shift FB" class="Bool (strict)"(error in=w942, "Value"=FALSE ("Mode Shift FB")) -> (error out=w940:errorcluster)  [unwired: 1 in, 1 out]
            n237 = property on="Temperature" class="Slide (strict)"(error in=w930, "Value"=2.5 ("Temperature")) -> (error out=w928:errorcluster)  [unwired: 1 in, 1 out]
            n238 = property on="Lid Status" class="Bool (strict)"(error in=w940, "Value"=FALSE ("Lid Status")) -> (error out=w938:errorcluster)  [unwired: 1 in, 1 out]
            n239 = property on="Pressure" class="Slide (strict)"(error in=w928, "Value"=0.0 ("Pressure")) -> (error out=w926:errorcluster)  [unwired: 1 in, 1 out]
          }
        }
        "DAQ Status" <- w459
        "DAQ On?" <- w457
        "Triac CW" <- w454
        "Traic CCW" <- w453
        "Cold Valve" <- w429
        "Recirc Pump" <- w430
        "Mode Shift" <- w416
        "Drain Pump" <- w431
        "Fabric SoftValve" <- w426
        "Spray/Rinse Valve" <- w427
        "Hot Valve" <- w428
        n240 = case shown="True" "MS (M - A)" {
          tunnel: w421 -> [w483 w494]
          tunnel: [w483 w493] -> w417
          tunnel: w416 -> [_ w484]
          frame False {
          }
          frame True {
            n241 = Equal?(x=w484, y=TRUE) -> (x = y?=w491:bool)
            n242 = case shown="True" w491 {
              tunnel: w494 -> [w499 w501]
              tunnel: [w499 w500] -> w486
              frame False {
              }
              frame True {
                n243 = Increment(x=w501) -> (x+1=w500:dbl)
              }
            }
            n244 = In Range and Coerce(upper limit=24.0, x=w486, lower limit=15.0) -> (In Range?=w488:bool)  [unwired: 1 out]
            n245 = case shown="True" w488 {
              frame False {
                n246 = property on="Mode Shift FB" class="Bool (strict)"("Value"=FALSE ("Mode Shift FB")) -> ()  [unwired: 2 in, 2 out]
              }
              frame True {
                n247 = property on="Mode Shift FB" class="Bool (strict)"("Value"=TRUE ("Mode Shift FB")) -> ()  [unwired: 2 in, 2 out]
              }
            }
            n248 = Greater Or Equal?(x=w486, y=24.0) -> (x >= y?=w485:bool)
            n249 = case shown="True" w485 {
              tunnel: w486 -> [w495 _]
              tunnel: [w495 0.0] -> w493
              frame False {
              }
              frame True {
              }
            }
          }
        }
        n250 = case shown="False" w424 {
          tunnel: w422 -> [w503 _]
          tunnel: [w502 0.0] -> w418
          frame False {
            n251 = Increment(x=w503) -> (x+1=w502:dbl)
          }
          frame True {
          }
        }
        n252 = Merge Errors(w468, w467, w466, w465, w464, w463, w462, w461, w460) -> (w469:errorcluster)
        n253 = call "Error_Control_Brass.vi"("Error In"=w469) -> ("Error Out"=w481:errorcluster)  [unwired: 14 in]
      }
      n254 = while "Periodic ERD Query Loop" {
        shift-right: [w186] -> w48
        shift-left: w75 -> [w188]
        tunnel: w65 -> [w189]
        shift-right: [w183] -> _
        shift-left: _ -> [w182]
        shift-right: [w177] -> _
        shift-left: w67 -> [w179]
        shift-right: [w172] -> _
        shift-left: _ -> [w171]
        tunnel: w63 -> [w170]
        tunnel: [w169] -> w46
        shift-right: [w168] -> _
        shift-left: _ -> [w167]
        tunnel: w59 -> [w166]
        i -> [w165]
        stop <- w185 stop-if-true
        # "ERD Loop"
        n255 = Dequeue Element(queue=w189, timeout in ms (-1)=0, error in (no error)=w188) -> (element=w174:T21, timed out?=w180:bool, error out=w187:errorcluster)  [unwired: 1 out]
        n256 = Unbundle By Name(w174) -> ("State"=w164:T22)
        n257 = Select(t=w179, s=w180, f=w164) -> (s? t:f=w178:T22)
        n258 = call "FGV_GEA2_Ref.vi"("Action"=enum16{"Set Ref", "Get Ref"}."Get Ref", "Error In"=w187) -> ("GEA2 Reference Out"=w173:refnum<k24>, "Error Out"=w176:errorcluster)  [unwired: 12 in]
        n259 = case shown="\"Read ERDs\"" w178 {
          tunnel: w176 -> [w199 w207 w220 w234 w253 w287 w333 w361 w369]
          tunnel: [w191 w203 w213 w234 w251 w286 w330 w361 w369] -> w184
          tunnel: [_ _ _ _ _ _ _ _ TRUE] -> w185
          tunnel: [w198 w205 w211 w237 w257 w280 w340 w362 w367] -> w183
          tunnel: w182 -> [w198 w205 w232 w237 w257 w280 w340 w362 w367]
          tunnel: T5 {"Source"=229, "Destination"=50} ("GEA Inputs") -> [_ _ w209 _ _ w284 _ _ _]
          tunnel: [ERD_Loop_States_Brass."Build ERD Read List" ("State") ERD_Loop_States_Brass."Read ERDs" ("State") ERD_Loop_States_Brass."Update UI" ("State") ERD_Loop_States_Brass."Update Graphs" ("State") ERD_Loop_States_Brass."Read Faults" ("State") ERD_Loop_States_Brass."Log Data" ("State") ERD_Loop_States_Brass."Read ERDs" ("State") ERD_Loop_States_Brass."Pause" ("State") ERD_Loop_States_Brass."Shutdown" ("State")] -> w177
          tunnel: w173 -> [_ _ w221 _ w246 w285 _ _ _]
          tunnel: [w196 w206 w210 w239 w255 w281 w339 w359 w365] -> w172
          tunnel: w171 -> [w196 _ w210 w239 w255 w281 w339 w359 w365]
          tunnel: w170 -> [w195 w202 w218 w235 w254 w279 w338 w358 w364]
          tunnel: [w195 w202 w218 w235 w254 w279 w337 w358 w364] -> w169
          tunnel: [w194 w201 w212 w236 w245 w282 w316 w357 w363] -> w168
          tunnel: w167 -> [w194 w201 _ w236 w243 w283 w316 w357 w363]
          tunnel: w166 -> [_ _ _ _ w247 _ _ _ _]
          tunnel: w165 -> [_ _ _ _ _ _ _ _ _]
          frame "Init", Default {
            # "Set Write Header\nFGV to True"
            n260 = call "Write_Header_FGV.vi"("Write Header ? In"=TRUE, "Action"=enum16{"Get", "Set"}."Set", "Error In"=w199) -> ("Error Out"=w191:errorcluster)  [unwired: 11 in, 1 out]
          }
          frame "Build ERD Read List" {
            n261 = call "ERD_Read_List_Builder.vi"("Array"="ERD Read List", "Error In"=w207) -> ("Read ERD List"=w206:T6[], "Error Out"=w203:errorcluster)  [unwired: 16 in]
          }
          frame "Read ERDs" {
            n262 = call "Convert Read ERD List to Message.vi"("GEA Inputs"=w209, "Read ERD List"=w210, "Error In"=w220) -> ("GEA Message"=w229:T3, "Error Out"=w230:errorcluster)  [unwired: 11 in]
            n263 = call "GEA2MessageFormatter.vi"("Prefix(Send/Recv)"="SEND", "GEA2 Data In"=w229, "Error In"=w230) -> ("Output String"=w228:string, "Error Out"=w227:errorcluster)  [unwired: 11 in]
            n264 = call "GExplorer_Queue_GEA2.vi"("Output String"=w228, "error in (no error)"=w227) -> ("error out"=w225:errorcluster)  [unwired: 13 in]
            n265 = Tick Count (ms)() -> (millisecond timer value=w211:u32)
            n266 = Subtract(x=w211, y=w232) -> (x-y=→"Log Rate (ms)":u32)
            n267 = call "GEA2 Read ERD Multiple Messages.vi"("GEA2 Reference In"=w221, "Retry Count"=2, "Read Timeout (ms)"=u32 500, "GEA Inputs"=w209, "Read ERD List"=w210, "Error In"=w225, "#ERDs per message"=6, "Verify ERD Response?"=FALSE) -> ("ERD Data Out"=w208:T30[], "Error Out"=w217:errorcluster)  [unwired: 4 in, 2 out]
            n268 = call "Write_Header_FGV.vi"("Action"=enum16{"Get", "Set"}."Get", "Error In"=w217) -> ("Write Header ? Out"=w214:bool, "Error Out"=w216:errorcluster)  [unwired: 12 in]
            n269 = call "Convert_ERDs_Brass.vi"("New Header?"=w214, "Array"=w208, "Error In"=w216) -> ("All_ERD_Data_Bundled_Brass"=w212:T31, "Error Out"=w213:errorcluster)  [unwired: 11 in]
          }
          frame "Update UI" {
            n270 = Unbundle By Name(w236) -> ("Version"=→"Version":T4, "ERD_Always Show"=→"ERD_Always Show":T1)
          }
          frame "Update Graphs" {
            n271 = case shown="True" "ERD Graphing ON" {
              tunnel: w253 -> [w269 w276]
              tunnel: [w269 w275] -> w252
              tunnel: "ERD Graph Cntrl" -> [_ w274]
              tunnel: [_ w273] -> w248
              tunnel: w246 -> [_ w272]
              tunnel: w243 -> [w268 w271]
              tunnel: [w268 w270] -> w242
              frame False {
              }
              frame True {
                n272 = call "Graph ERD Read List_Brass.vi"("GEA2 Reference In"=w272, "All_Bundled_Data_Brass"=w271, "ERD Graph Cntrl"=w274, "Error In"=w276) -> ("ERD Graph  Ind"=w273:T9, "All_Bundled_Data_Brass 2"=w270:T31, "Error Out"=w275:errorcluster)  [unwired: 8 in, 1 out]
              }
            }
            n273 = case shown="True" "Graphing ON" {
              tunnel: w252 -> [w258 w267]
              tunnel: [w258 w266] -> w251
              tunnel: w248 -> [_ w264]
              tunnel: w247 -> [_ _]
              tunnel: w242 -> [w259 w260]
              tunnel: [w259 w260] -> w245
              frame False {
              }
              frame True {
                n274 = call "Update Graphs_Brass.vi"("Select Graph"="Select Graph", "ERD Graph  Ind 2"=w264, "Error In"=w267) -> ("ERD 3"=→"ERD 3":dbl, "ERD 2"=→"ERD 2":dbl, "ERD 1"=→"ERD 1":dbl, "Error Out"=w266:errorcluster)  [unwired: 9 in]
                "ERD Graph  Ind" <- w264
              }
            }
          }
          frame "Read Faults" {
            n275 = case shown="True" "Fault ON" {
              tunnel: w287 -> [w288 w296]
              tunnel: [w288 w295] -> w286
              tunnel: w285 -> [_ w294]
              tunnel: w284 -> [_ w293]
              tunnel: w283 -> [w289 w292]
              tunnel: [w289 w291] -> w282
              frame False {
              }
              frame True {
                # "0-11 Sequence\n12-19 Table"
                n276 = call "GEA2 Read ERD Multiple Messages.vi"("GEA2 Reference In"=w294, "Read Timeout (ms)"=u32 500, "GEA Inputs"=w293, "Read ERD List"=T6[] [{"ERD Number"=132, "Data Type"=enum."string"}, {"ERD Number"=141, "Data Type"=enum."uint32_t"}, {"ERD Number"=57394, "Data Type"=enum."string"}, {"ERD Number"=57395, "Data Type"=enum."string"}, {"ERD Number"=57396, "Data Type"=enum."string"}, {"ERD Number"=57397, "Data Type"=enum."string"}, {"ERD Number"=57398, "Data Type"=enum."string"}, {"ERD Number"=57399, "Data Type"=enum."string"}, {"ERD Number"=57400, "Data Type"=enum."string"}, {"ERD Number"=57401, "Data Type"=enum."string"}, {"ERD Number"=57402, "Data Type"=enum."string"}, {"ERD Number"=57403, "Data Type"=enum."string"}, {"ERD Number"=129, "Data Type"=enum."string"}, {"ERD Number"=57444, "Data Type"=enum."string"}, {"ERD Number"=57445, "Data Type"=enum."string"}, {"ERD Number"=57446, "Data Type"=enum."string"}, {"ERD Number"=57447, "Data Type"=enum."string"}, {"ERD Number"=57448, "Data Type"=enum."string"}, {"ERD Number"=57449, "Data Type"=enum."string"}, {"ERD Number"=57450, "Data Type"=enum."string"}], "Error In"=w296, "#ERDs per message"=4 ("#ERDs per message 2"), "Verify ERD Response?"=FALSE) -> ("ERD Data Out"=w301:T30[], "Error Out"=w295:errorcluster)  [unwired: 5 in, 2 out]
                n277 = Array Subset(array=w301, index=12, length=8) -> (w302:T30[])
                n278 = Array Subset(array=w301, index=0, length=12) -> (w300:T30[])
                n279 = call "Fault_Table_Read.vi"("ERD Data Out"=w302) -> ("Fault Set?"=→"Fault Status":bool, "Table Buffer Status"=→"Table Buffer Status":T13, "Fault Table String Out"=→"Fault Table Buffer":string[][], "Fault Table Array Out"=w290:T33)  [unwired: 11 in]
                n280 = call "Fault_Seq_Read.vi"("Seq ERD In"=w300) -> ("Seq Buffer Status"=→"Seq Buffer Status":T13, "String"=→"Fault Sequence Buffer":string)  [unwired: 13 in]
                n281 = Bundle By Name(cluster=w292, "Fault Table Array"=w290) -> (w291:T31)
              }
            }
          }
          frame "Log Data" {
            # "TimeStamp"
            # "Append With Fault Log Data"
            # "Write Date/Time Header"
            n282 = Unbundle By Name(w316) -> ("CSV File String Arrays.ERD Name Array"=w336:string[], "CSV File String Arrays.ERD Number Array"=w335:string[], "CSV File String Arrays.ERD Converted String Data"=w328:string[])
            n283 = call "Write_Header_FGV.vi"("Action"=enum16{"Get", "Set"}."Get", "Error In"=w333) -> ("Write Header ? Out"=w314:bool, "Error Out"=w327:errorcluster)  [unwired: 12 in]
            n284 = case shown="True" w314 {
              tunnel: w336 -> [w349 _]
              tunnel: [w351 string[] [] ("ERD Name Array")] -> w326
              tunnel: w335 -> [w350 _]
              tunnel: [w354 string[] [] ("ERD Number Array")] -> w324
              frame True {
                n285 = Insert Into Array(array=w350, index=0, new element #1="", new element #2="", new element #3="", new element #4="") -> (w354:string[])
                n286 = Insert Into Array(array=w349, index=0, new element #1="Date", new element #2="Time", new element #3="HH:MM:SS", new element #4=".SS" ("new element/subarray")) -> (w351:string[])
              }
              frame False {
              }
            }
            n287 = call "TimeStamp to String Array.vi"("String Array In"=w328) -> ("String Array Out"=w322:string[])  [unwired: 10 in]
            n288 = Unbundle By Name(w316) -> ("Fault Table Array"=w315:T33)
            n289 = call "Faults_To_String_Array.vi"("Write Header ?"=w314, "Fault Table Entry"=w315, "Error In"=w327) -> ("Fault Header String Array"=w321:string[], "Fault ERD Number String Array"=w320:string[], "Fault Data String Array"=w319:string[], "Error Out"=w317:errorcluster)  [unwired: 13 in]
            n290 = Insert Into Array(array=w326, new element=w321) -> (w325:string[])  [unwired: 1 in]
            n291 = Insert Into Array(array=w324, new element=w320) -> (w323:string[])  [unwired: 1 in]
            n292 = Insert Into Array(array=w322, new element=w319) -> (w318:string[])  [unwired: 1 in]
            n293 = call "Write _To_CSV_File.vi"("Refnum In"=w338, "String Array 1"=w325, "String Array 2"=w323, "String Array 3"=w318, "Error In"=w317) -> ("Refnum Out"=w337:refnum<file>, "Error Out"=w331:errorcluster)  [unwired: 12 in, 1 out]
            n294 = call "Write_Header_FGV.vi"("Write Header ? In"=FALSE, "Action"=enum16{"Get", "Set"}."Set", "Error In"=w331) -> ("Error Out"=w330:errorcluster)  [unwired: 11 in, 1 out]
          }
          frame "Pause" {
          }
          frame "Shutdown" {
          }
        }
        n295 = call "Error_Control_Brass.vi"("Error In"=w184) -> ("Error Out"=w186:errorcluster)  [unwired: 14 in]
      }
      n296 = while "GEA2 Receive Message Loop" {
        shift-right: [w1213] -> w125
        shift-left: w31 -> [w1214]
        shift-right: [w1210] -> _
        shift-left: w114 -> [w1215]
        stop <- w1212 stop-if-true
        # "GEA2 Receive Message Loop"
        n297 = event shown="[0] <Data>: User Event" {
          selector: w1215 -> [w1231 w1233 w1249 w1255]
          dyn-events: [w1231 w1233 w1244 w1255] -> w1210
          timeout: _ -> [_ _ _ _]
          tunnel: w1214 -> [w1230 w1235 w1252 w1257]
          tunnel: [w1218 w1235 w1237 w1257] -> w1211
          tunnel: [FALSE TRUE _ TRUE] -> w1212
          event User Event {
            n298 = event-data() -> ("Source"=w1225:u8, "Destination"=w1224:u8, "Command"=w1223:u8, "Message"=w1222:string)  [unwired: 1 in]
            n299 = Bundle By Name(cluster=T3 {"Source"=0, "Destination"=0, "Command"=0, "Message"=""} ("GEA2 Msg"), "Source"=w1225, "Destination"=w1224, "Command"=w1223, "Message"=w1222) -> (w1216:T3)
            n300 = call "GEA2 Log Filter.vi"("Filter Log"="Filter Log", "Filter Data"="Filter Data", "GEA2 Msg"=w1216, "Cmd to Filter"="Cmd", "error in (no error)"=w1230) -> ("error out"=w1219:errorcluster)  [unwired: 10 in]
            n301 = call "FGV_GEA2_Ref.vi"("Action"=enum16{"Set Ref", "Get Ref"}."Get Ref", "Error In"=w1219) -> ("GEA2 Reference Out"=w1217:refnum<k24>, "Error Out"=w1220:errorcluster)  [unwired: 12 in]
            n302 = call "ACK Subscriptions Publications.vi"("GEA2 Reference In"=w1217, "GEA2 Msg"=w1216, "error in (no error)"=w1220) -> ("error out"=w1218:errorcluster)  [unwired: 11 in, 1 out]
          }
          event User Event {
            n303 = event-data() -> ()  [unwired: 1 in, 1 out]
          }
          event "Board Index": Value Change {
            # "Stop old GEA2\nbus reference"
            # "Allow other references a chance\nto begin using new reference"
            # "Store new GEA2 bus reference"
            # "Update event registration\nand initialize new GEA2 bus"
            # "Get the previous GEA2\nbus ref, but don't stop it\nuntil we update the FGV\nwith the new GEA2 ref"
            n304 = event-data() -> ("NewVal"=w1248:u8)  [unwired: 1 in]
            n305 = property on="Board Index" class="DigNum (strict)"(error in=w1252, "DisabledEnum"=T28."Disabled and Grayed Out" ("Disabled")) -> (error out=w1253:errorcluster)  [unwired: 1 in, 1 out]
            n306 = call "FGV_GEA2_Ref.vi"("Action"=enum16{"Set Ref", "Get Ref"}."Get Ref", "Error In"=w1253) -> ("GEA2 Reference Out"=w1236:refnum<k24>, "Error Out"=w1250:errorcluster)  [unwired: 12 in]
            n307 = call "GEA2_Reregister.vi"("Board Index"=w1248, "Event Registration In"=w1249, "Error In"=w1250) -> ("GEA2 Reference Out"=w1242:refnum<k24>, "Board ID"=w1245:string, "Event Registration Out"=w1244:refnum<event-registration>, "Error Out"=w1246:errorcluster)  [unwired: 9 in]
            n308 = property on="Board Index" class="DigNum (strict)"(error in=w1246, "DisabledEnum"=T28."Enabled" ("Disabled")) -> (error out=w1243:errorcluster)  [unwired: 1 in, 1 out]
            n309 = local write "Board ID"(w1245) -> ()
            n310 = call "FGV_GEA2_Ref.vi"("GEA2 Reference In"=w1242, "Action"=enum16{"Set Ref", "Get Ref"}."Set Ref", "Error In"=w1243) -> ("Error Out"=w1239:errorcluster)  [unwired: 11 in, 1 out]
            n311 = call "Time Delay"("error in (no error)"=w1239, "Delay Time (s)"=3.0) -> ("error out"=w1238:errorcluster)  [unwired: 9 in]
            n312 = call "GEA2 Stop.vi"("GEA2 Reference In"=w1236, "Error In"=w1238) -> ("Error Out"=w1237:errorcluster)  [unwired: 13 in]
          }
          event "Stop": Value Change {
            n313 = event-data() -> ()  [unwired: 1 in, 6 out]
          }
        }
        n314 = call "Error_Control_Brass.vi"("Error In"=w1211) -> ("Error Out"=w1213:errorcluster)  [unwired: 14 in]
      }
      n315 = while "Continuous Send Loop" {
        shift-right: [w139] -> _
        shift-left: Cont_Send_States."Run" ("State") -> [w138]
        tunnel: w36 -> [w140]
        tunnel: [w133] -> _
        shift-right: [w131] -> w40
        shift-left: w31 -> [w142]
        stop <- w141 stop-if-true
        # "Continuous Send Loop"
        n316 = Dequeue Element(queue=w140, timeout in ms (-1)=0, error in (no error)=w142) -> (queue out=w134:refnum<queue>, element=w127:T17, timed out?=w135:bool, error out=w130:errorcluster)
        n317 = Select(t=w138, s=w135, f=w127) -> (s? t:f=w137:T17)
        n318 = property on="GEA2 Send" class="Clust (strict)"() -> ("Value"=w129:T3)  [unwired: 2 in, 2 out]
        n319 = case shown="\"Run\", Default" w137 {
          selector: w137 -> [w146 w161]
          tunnel: w130 -> [w148 w163]
          tunnel: [w147 w163] -> w132
          tunnel: [_ TRUE] -> w141
          tunnel: [w146 w161] -> w139
          tunnel: w134 -> [w145 w160]
          tunnel: [w145 w160] -> w133
          tunnel: w129 -> [w144 _]
          frame "Run", Default {
            n320 = case shown="True" "Start Send" {
              tunnel: w148 -> [w149 w152]
              tunnel: [w149 w156] -> w147
              tunnel: w144 -> [_ w154]
              frame False {
              }
              frame True {
                n321 = call "FGV_GEA2_Ref.vi"("Action"=enum16{"Set Ref", "Get Ref"}."Get Ref", "Error In"=w152) -> ("GEA2 Reference Out"=w150:refnum<k24>, "Error Out"=w151:errorcluster)  [unwired: 12 in]
                n322 = call "GEA2MessageFormatter.vi"("Prefix(Send/Recv)"="SEND", "GEA2 Data In"=w154, "Error In"=w151) -> ("Output String"=w155:string, "Error Out"=w159:errorcluster)  [unwired: 11 in]
                n323 = call "GExplorer_Queue_GEA2.vi"("Output String"=w155, "error in (no error)"=w159) -> ("error out"=w157:errorcluster)  [unwired: 13 in]
                n324 = call "GEA2 Send Message.vi"("GEA2 Reference In"=w150, "Input Data"=w154, "Error In"=w157) -> ("Error Out"=w156:errorcluster)  [unwired: 11 in, 1 out]
              }
            }
          }
          frame "Shutdown" {
          }
        }
        n325 = call "Error_Control_Brass.vi"("Error In"=w132) -> ("Error Out"=w131:errorcluster)  [unwired: 14 in]
        n326 = Wait (ms)(milliseconds to wait="Msg Rate (ms)") -> ()  [unwired: 1 out]
      }
      n327 = while "GEA2 Display Loop" {
        tunnel: w66 -> [w379]
        shift-right: [w376] -> _
        shift-left: _ -> [w382]
        shift-right: [w378] -> w95
        shift-left: w30 -> [w386]
        tunnel: w28 -> [w372]
        tunnel: [w370] -> w26
        stop <- w380 stop-if-true
        # "GEA2 Display Loop"
        n328 = Dequeue Element(queue=w379, error in (no error)=w386) -> (element=w385:T19, error out=w381:errorcluster)  [unwired: 1 in, 2 out]
        n329 = Unbundle By Name(w385) -> ("Data"=w383:variant, "State"=w384:enum16{"Add to Log", "Clear", "Shutdown"})
        n330 = case shown="\"Add to Log\", Default" w384 {
          tunnel: w383 -> [w397 _ _]
          tunnel: w382 -> [w400 w405 _]
          tunnel: [w399 w405 ""] -> w377
          tunnel: w381 -> [w398 w406 w410]
          tunnel: [w395 w406 w410] -> w373
          tunnel: [FALSE TRUE FALSE] -> w380
          tunnel: [w387 _ _] -> w371
          frame "Add to Log", Default {
            n331 = Variant To Data(error in=w398, type="", Variant=w397) -> (data=w389:string, error out=w395:errorcluster)
            n332 = String Subset(string=w389, offset (0)=22, length (rest)=7 ("length (rest)")) -> (substring=w390:string)
            n333 = Equal?(x="SEND E5", y=w390) -> (x = y?=w388:bool)
            n334 = case shown="True" w388 {
              tunnel: w400 -> [w403 w404]
              tunnel: [w402 w404] -> w399
              tunnel: w389 -> [w401 _]
              tunnel: [w401 _] -> w387
              frame False {
                n335 = Concatenate Strings(w401, w403) -> (w402:string)
              }
              frame True {
              }
            }
          }
          frame "Shutdown" {
          }
          frame "Clear" {
          }
        }
        "GEA2 Log" <- w377
        n336 = call "Write _To_TXT_File.vi"("refnum"=w372, "text"=w371, "error in"=w373) -> ("refnum out"=w370:refnum<file>, "error out"=w374:errorcluster)  [unwired: 10 in, 1 out]
        n337 = call "Error_Control_Brass.vi"("Error In"=w374) -> ("Error Out"=w378:errorcluster)  [unwired: 14 in]
        n338 = String Subset(string=w377, length (rest)="GEA2 Log Length") -> (substring=w376:string)  [unwired: 1 in]
      }
      n339 = Close File(refnum=w26, error in=w95) -> (error out=w27:errorcluster)  [unwired: 1 out]
      n340 = call "GEA2 Stop.vi"("GEA2 Reference In"=w123, "Error In"=w124) -> ("Error Out"=w107:errorcluster)  [unwired: 13 in]
      n341 = Close File(refnum=w46, error in=w48) -> (error out=w47:errorcluster)  [unwired: 1 out]
      n342 = Merge Errors(w47, w27, w40, w125, w107, w94) -> (w22:errorcluster)
      n343 = Obtain Queue(name (unnamed)="Continuous Send", element data type=Cont_Send_States_Brass."Run" ("State"), error in (no error)=w22) -> (queue out=w45:refnum<queue>, error out=w44:errorcluster)  [unwired: 2 in, 1 out]
      n344 = Obtain Queue(name (unnamed)="ERD Loop", element data type=T21 {"Data"=variant, "State"=enum."Read ERDs"} ("Data"), error in (no error)=w22) -> (queue out=w102:refnum<queue>, error out=w101:errorcluster)  [unwired: 2 in, 1 out]
      n345 = Obtain Queue(name (unnamed)="GEA2", element data type=T19 {"Data"=variant, "State"=enum."Add to Log"} ("Data"), error in (no error)=w22) -> (queue out=w111:refnum<queue>, error out=w110:errorcluster)  [unwired: 2 in, 1 out]
      n346 = Obtain Queue(name (unnamed)="DAQ", element data type=DAQ_States_Brass."Wait for Init" ("States"), error in (no error)=w22) -> (queue out=w97:refnum<queue>, error out=w98:errorcluster)  [unwired: 2 in, 1 out]
      n347 = Release Queue(queue=w45, error in (no error)=w44) -> (error out=w43:errorcluster)  [unwired: 1 in, 2 out]
      n348 = Release Queue(queue=w102, error in (no error)=w101) -> (error out=w90:errorcluster)  [unwired: 1 in, 2 out]
      n349 = Release Queue(queue=w111, error in (no error)=w110) -> (error out=w91:errorcluster)  [unwired: 1 in, 2 out]
      n350 = Release Queue(queue=w97, error in (no error)=w98) -> (error out=w92:errorcluster)  [unwired: 1 in, 2 out]
      n351 = Merge Errors(w43, w90, w91, w92) -> (w89:errorcluster)
      n352 = call "Error_Control_Brass.vi"("Command (Handle Errors)"=Error_Command_Brass."Report Errors", "Error In"=w89) -> ("Error Out"=w82:errorcluster)  [unwired: 13 in]
    }
    frame Error {
    }
  }
  n353 = call <vilib>:"Simple Error Handler.vi"("error in (no error)"=w2) -> ("error out"=→"Error Out":errorcluster)  [unwired: 4 in, 4 out]
